vi "MegaAwesome_12_09_14b_PD(testing).vi"() -> ()   [LabVIEW 2012]
uses:
  data/MegaAwesome_States.ctl
  <vilib>/Utility/inputDevices.llb/keyboardAcquire.vi
  <vilib>/Utility/file.llb/Write To Spreadsheet File (string).vi
  <vilib>/Utility/file.llb/Read From Spreadsheet File (string).vi
panel:
  out "Vd_Sat":dbl
  in  "Vd_Sat Index":i32=2
  in  "Vd_Lin Index":i32=1
  out "Stats Label":string
  in  "Disable Flag 2":bool caption="Disable Flag"
  out "Save Next?":bool
  out "Image Center X":i32
  in  "Disable Flag":bool
  out "Index":string
  out "Opj X Axis":string
  out "X Axis Display Type":string
  in  "Index-Sat":dbl=5.0
  in  "Index-Lin":dbl=5.0
  in  "IndexLog-Lin":dbl=5.0
  in  "IndexLog-Sat":dbl=5.0 caption="Num Pts"
  out "Lin Id-Log Used":dbl[](array[numeric])
  out "Lin-Vg Array-Log Used":dbl[](array[numeric])
  out "Save Array":string[][](array[string])
  out "Folder Index":i32 caption="Length"
  out "Sat Id-Used":dbl[](array[numeric])
  out "Sat Vg Array-Used":dbl[](array[numeric])
  out "Vg Array-Log-Used":dbl[](array[numeric])
  out "Sat Id-Log-Used":dbl[](array[numeric])
  out "Lin Id-Used":dbl[](array[numeric])
  out "Lin-Vg Array-Used":dbl[](array[numeric])
  out "Lin Vd":dbl
  out "Recorded Prop":T1
  out "Current State":T2=enum."File Missing"
  in  "Main Tab Control":T3(tab)
  in  "LKG (TRF) Folder":path caption="Folder"
  out "LKG (TRF) File":path caption="File File"
  in  "Transfer File":path
  out "Transfer Folder":path
  in  "Transport\nFolder":path caption="Transport Folder"
  out "Transport\nFile":path caption="Transport File"
  in  "Image Folder":path
  out "Image File":path
  out "Fabrication Prop":T4
  out "Distances":i32[](array[numeric])
  in  "Zoom":i32(slide)=-3 scale=-5.0..5.0
  in  "Magnification":i32(ring) items=["5x", "10x", "20x", "50x", "80x"]
  in  "Undo Button":bool
  in  "Remove Button":bool
  in  "Transfer Plots":T5(tab)=enum."Saturation"
  in  "Lin-Trans Slider":dbl(slide) step=1.0 scale=0.0..61.0 scale format="%#_2p"
  out "Sqrt-Lin":cluster{dbl[], dbl[]}[](graph)
  in  "Sat-Trans Slider":dbl(slide) min=0.0 max=162.0 step=1.0 scale=0.0..61.0 scale format="%#_2p"
  out "Sqrt-Sat":cluster{dbl[], dbl[]}[](graph)
  out "Used Vg \nSqrt Sat":dbl
  out "Raw- Lin":cluster{dbl[], dbl[]}[](graph)
  out "Raw- Sat":cluster{dbl[], dbl[]}[](graph)
  in  "Log Plots":T6(tab)=enum."Saturation"
  in  "Lin-Log Slider":dbl(slide) step=1.0 scale=0.0..61.0 scale format="%#_1p"
  out "Lin-Log":cluster{dbl[], dbl[]}[](graph)
  out "Used Vg \nLog Lin":dbl
  in  "Sat-Log Slider":dbl(slide) step=1.0 scale=0.0..61.0 scale format="%#_1p"
  out "Sat-Log":cluster{dbl[], dbl[]}[](graph)
  out "Used Vg \nLog Sat":dbl
  out "Transport":cluster{ext[], ext[]}[](graph)
  out "Transport Name:":string
  out "LKG (TSF)":cluster{ext[], ext[]}[](graph)
  out "LKG (TRF) Name":string
  in  "Manual Controls":T7
  in  "File Controls":T8
  out "Date Recorded":string="Date Recorded" caption="Measured"
  out "Data Name:":string
  out "Image Name":string
  out "Date Created":string caption="Fabricated"
  in  "Comments:":string
  out "Rec: Length":dbl caption="Length"
  out "Rec: Width":dbl caption="Width"
  out "Rec: Dielectric (d)":dbl caption="Dielectric (d)" format="%#_3g"
  in  "New: Dielectric":dbl
  in  "New: Length":dbl
  in  "New: Width":dbl
  out "Rec: Temp":dbl caption="Sample Temp" format="%.1f"
  in  "New: Temp":dbl format="%.1f"
  out "Image Out":T9(plugin-control)
  in  "Num Pts":i32=5
  in  "Num Pts Log":i32=5 caption="Num Pts"
  out "Recorded Values Cluster":T10
  out "Calculated Values Cluster":T10 caption="Recorded Values Cluster"
  out "Re-Calculated Values Cluster":T10 caption="Recorded Values Cluster"
  in  "Independant Variable:":string(combo)="Length (um):"
  out "Image Preview":T9(plugin-control)
  out "Total Width":i32
  in  "Index Array":i32(ring) caption="Index" items=["2M", "2N", "2O", "2P", "3M", "3N", "3O", "3P"]
  in  "Hysteresis Analysis":enum32{"1st Sweep", "2nd Sweep", "Both"}(radio)
  in  "Dielectric Constant":dbl=3.9
  in  "Scale Factors":T11={"5x"=0.5495, "10x"=0.2755, "20x"=0.1389, "50x"=0.0546, "80x"=0.0337}
  in  "Room Temp":dbl=294.0 caption="Room Temp (K)"
  out "No Image\n File":path=path "\\\\acad1\\physics/Jurchescu-group/JW-PD/Mega Awesome/data/Image Not Found.png" caption="No Image File"
  out "Origin Project File":path=path "\\\\acad1\\physics/Jurchescu-group/JW-PD/Mega Awesome/data/Origin Template.opj"
  out "No Transport\n File":path=path "\\\\acad1\\physics/Jurchescu-group/JW-PD/Mega Awesome/data/No Transport File.txt" caption="No Transport File"
  in  "Transport Style Controls":T12={"Transport Line Size"=1, "Transport Line Color"=16772608} {"Transport Line Size" items=["Extra Small", "Small", "Medium", "Large", "Extra Large"]}
  out "Application Directory":path=path "\\\\acad1\\physics/Jurchescu-group/JW-PD/Mega Awesome"
  in  "LKG Style Controls":T13={"Transport Line Size"=1, "LKG (TRF) Line Color"=16772608} {"Transport Line Size" items=["Extra Small", "Small", "Medium", "Large", "Extra Large"]}
  out "Progress":i32(slide) max=46 step=1 scale=0.0..100.0
  # "1)  Select the Transfer File that you would like to analyze:"
  # "Transfer Location"
  # "2) What else would you like to view during your analysis?"
  # "Transport Location"
  # "Image Location"
  # "Gate Leakge (TRF) Location"
  # "Recorded"
  # "Calculated"
  # "Re-Calculated"
  # "Manual"
  # "um"
  # "V"
  # "V"
  # "V"
  # "Default File Choices"
  # "Scale Factors"
  # "Default Analysis Values"
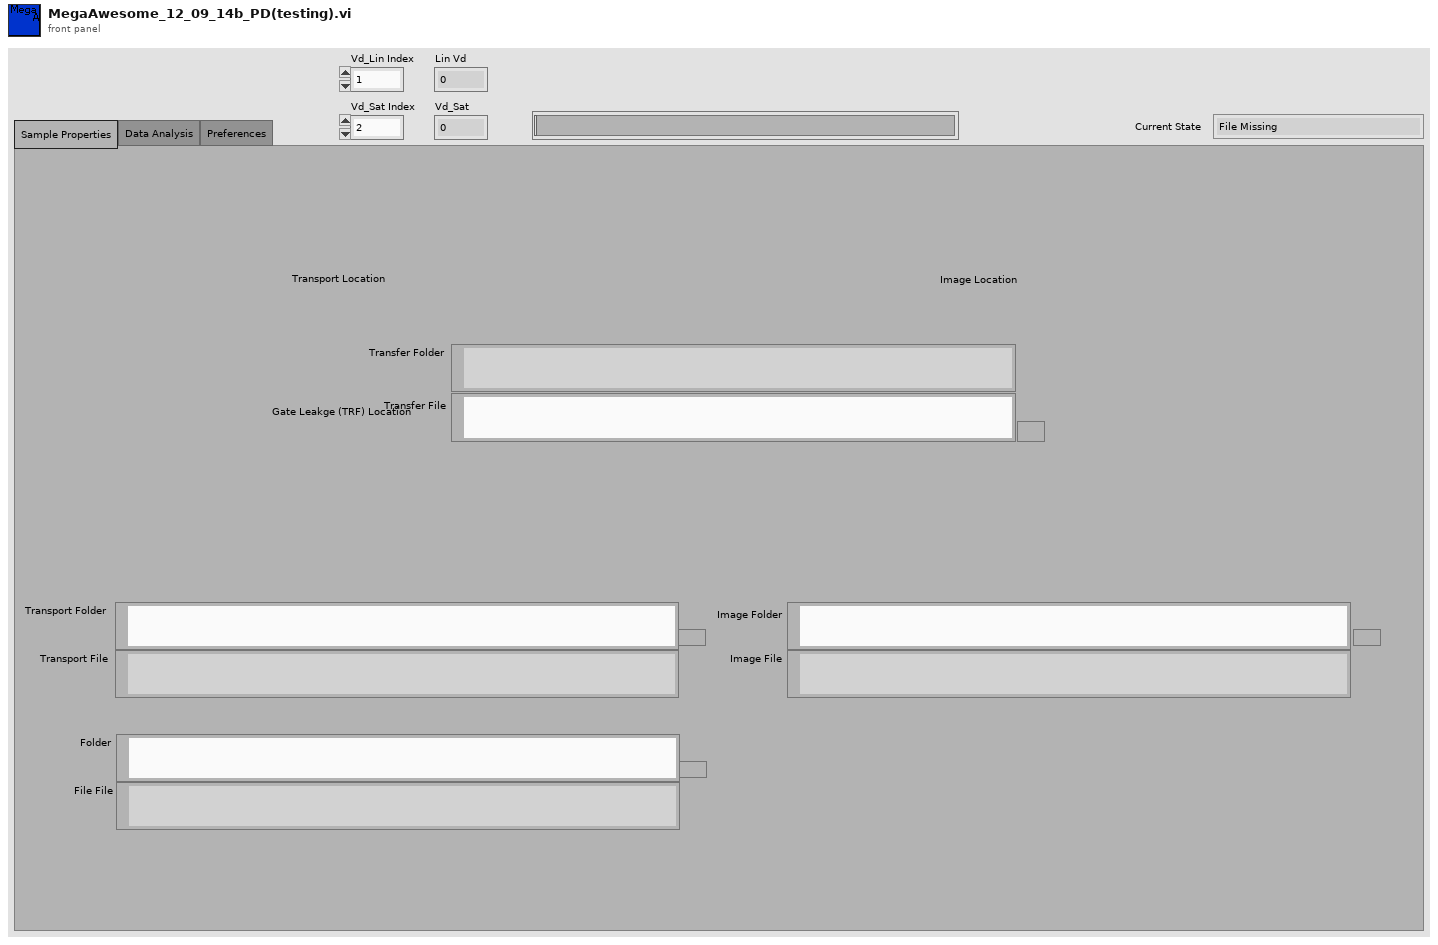
[diagram p1: front panel]
types:
  T1 = cluster{"Date Recorded":string, "Index":string, "Length":dbl, "Width":dbl, "Sample Temp":dbl}
  T2 = typedef "MegaAwesome_States.ctl" = enum16{"Init", "File Missing", "No Event", "Read Data", "Calculated Values", "Re-Calculated Values", "Next File", "Previous File", "Discard File", "Save", "Save Lines", "Export", "Exit"}
  T3 = enum32{"Sample Properties", "Data Analysis", "Preferences"}
  T4 = cluster{"Date Created":string, "Material":string, "Solvent":string, "Concentration":dbl, "Method":string, "Dielectric (nm)":dbl, "Treatment":string, "Comments":string}
  T5 = enum32{"Linear", "Saturation", "Raw-Linear", "Raw-Saturation"}
  T6 = enum32{"Linear", "Saturation", "Transport", "Gate Current (TSF)"}
  T7 = cluster{"Manual-Temp":bool, "Manual-Width":bool, "Manuel-Length":bool, "Manuel-Dielectric":bool, "Manual Comments":bool}
  T8 = cluster{"Previous File":bool, "Discard ":bool, "Save Lines":bool, "Close":bool, "Next File ":bool, "Save":bool, "Save Next":bool, "Export":bool}
  T9 = typedef "IMAQ Image.ctl" = refnum<image>
  T10 = cluster{"Mobility-Sat":dbl, "Moblitity-Lin":dbl, "On/Off":dbl, "Off Current":dbl, "Vt-Sat":dbl, "STS":dbl, "Trap Density-VT":dbl, "Trap Density-STS":dbl}
  T11 = cluster{"5x":dbl, "10x":dbl, "20x":dbl, "50x":dbl, "80x":dbl}
  T12 = cluster{"Transport Line Size":u16, "Transport Line Color":u32}
  T13 = cluster{"Transport Line Size":u16, "LKG (TRF) Line Color":u32}
  T14 = enum8{"Enabled", "Disabled", "Disabled and Grayed Out"}
  T15 = typedef "LVBoundsTypeDef.ctl" = cluster{"Width":u32, "Height":u32}
  T16 = enum16{"0", "1", "2", "3", "4", "5", "6", "7", "8", "9", "A", "B", "C", "D", "E", "F", "G", "H", "I", "J", "K", "L", "M", "N", "O", "P", "Q", "R", "S", "T", "U", "V", "W", "X", "Y", "Z", "F1", "F2", "F3", "F4", "F5", "F6", "F7", "F8", "F9", "F10", "F11", "F12", "F13", "F14", "F15", "ADD", "BACK", "BACKSLASH", "CAPITAL", "COMMA", "DECIMAL", "DELETE", "DIVIDE", "DOWN", "END", "EQUALS", "ESCAPE", "GRAVE (`)", "HOME", "INSERT", "LBRACKET", "LCONTROL", "LEFT", "L ALT", "LSHIFT", "LWIN", "MINUS", "MULTIPLY", "NEXT", "NUMLOCK", "NUMPAD_0", "NUMPAD_1", "NUMPAD_2", "NUMPAD_3", "NUMPAD_4", "NUMPAD_5", "NUMPAD_6", "NUMPAD_7", "NUMPAD_8", "NUMPAD_9", "PAUSE", "PERIOD", "PRIOR (PG UP)", "RBRACKET", "RCONTROL", "RETURN", "RIGHT", "R ALT", "RSHIFT", "RWIN", "SCROLL", "SEMICOLON", "SLASH", "SPACE", "SUBTRACT", "TAB", "UP", "ENTER (num pad)", "' (quote)"}[]
  T17 = enum16{"0", "1", "2", "3", "4", "5", "6", "7", "8", "9", "A", "B", "C", "D", "E", "F", "G", "H", "I", "J", "K", "L", "M", "N", "O", "P", "Q", "R", "S", "T", "U", "V", "W", "X", "Y", "Z", "F1", "F2", "F3", "F4", "F5", "F6", "F7", "F8", "F9", "F10", "F11", "F12", "F13", "F14", "F15", "ADD", "BACK", "BACKSLASH", "CAPITAL", "COMMA", "DECIMAL", "DELETE", "DIVIDE", "DOWN", "END", "EQUALS", "ESCAPE", "GRAVE (`)", "HOME", "INSERT", "LBRACKET", "LCONTROL", "LEFT", "L ALT", "LSHIFT", "LWIN", "MINUS", "MULTIPLY", "NEXT", "NUMLOCK", "NUMPAD_0", "NUMPAD_1", "NUMPAD_2", "NUMPAD_3", "NUMPAD_4", "NUMPAD_5", "NUMPAD_6", "NUMPAD_7", "NUMPAD_8", "NUMPAD_9", "PAUSE", "PERIOD", "PRIOR (PG UP)", "RBRACKET", "RCONTROL", "RETURN", "RIGHT", "R ALT", "RSHIFT", "RWIN", "SCROLL", "SEMICOLON", "SLASH", "SPACE", "SUBTRACT", "TAB", "UP", "ENTER (num pad)", "' (quote)"}
  T18 = typedef "ROI Descriptor" = cluster{"Global Rectangle":i32[], "Contours":cluster{"ID":enum32{"External", "Internal"}, "Type":u32, "Coordinates":i32[]}[]}
  T19 = cluster{string, sgl, bool, bool, bool, bool, bool, bool, i32}
  T20 = cluster{i32, cluster{string, sgl, bool, bool, bool, bool, bool, bool, i32}, i32, i32}
  T21 = cluster{"Global Rectangle":i32[], "Contours":cluster{"Contour Type":u32, "ROI Type":u32, "Points":i32[]}[]}
  T22 = cluster{"Contour Type":u32, "ROI Type":u32, "Points":i32[]}[]
  T23 = cluster{"[0]":cluster{dbl[], dbl[]}, "[1]":cluster{dbl[], dbl[]}, "[2]":cluster{dbl[], dbl[]}, "[3]":cluster{dbl[], dbl[]}, "[4]":cluster{dbl[], dbl[]}, "[5]":cluster{dbl[], dbl[]}, "[6]":cluster{dbl[], dbl[]}, "[7]":cluster{dbl[], dbl[]}, "[8]":cluster{dbl[], dbl[]}}
  T24 = cluster{i32[], cluster{"Contour Type":u32, "ROI Type":u32, "Points":i32[]}[]}
  T25 = cluster{"Contour Type":u32, "ROI Type":u32, "Points":i32[]}
  T26 = cluster{"Points[0]":i32, "Points[1]":i32, "Points[2]":i32, "Points[3]":i32, "Points[4]":i32, "Points[5]":i32, "Points[6]":i32, "Points[7]":i32, "Points[8]":i32}
  T27 = cluster{"Sat Vg Used":dbl[], "Sat Sqrt(Id) Used ":dbl[], "Lin Vg Used":dbl[], "Lin Sqrt(Id) Used":dbl[], "Index-Lin":dbl, "Index-Sat":dbl}
  T28 = cluster{"Raw Sat":cluster{dbl[], dbl[]}[], "Sqrt Sat":cluster{dbl[], dbl[]}[], "Log Sat":cluster{dbl[], dbl[]}[], "Raw Lin":cluster{dbl[], dbl[]}[], "Sqrt Lin":cluster{dbl[], dbl[]}[], "Log Lin":cluster{dbl[], dbl[]}[]}
  T29 = cluster{"Mobility-Sat":dbl, "Vt-Sat":dbl, "Mobility-Lin":dbl, "Vt-Lin":dbl, "Off I-Sat":dbl, "On/Off I-Sat":dbl}
  T30 = cluster{"Sat Vg Used":dbl[], "Sat Log(Id) Used":dbl[], "Lin Vg Used":dbl[], "Lin Log(Id) Used":dbl[], "STS Index-Sat":dbl, "STS Index-Lin":dbl}
  T31 = cluster{"Independant  Variable Indicator":string, "Parameter String Indicator":string}
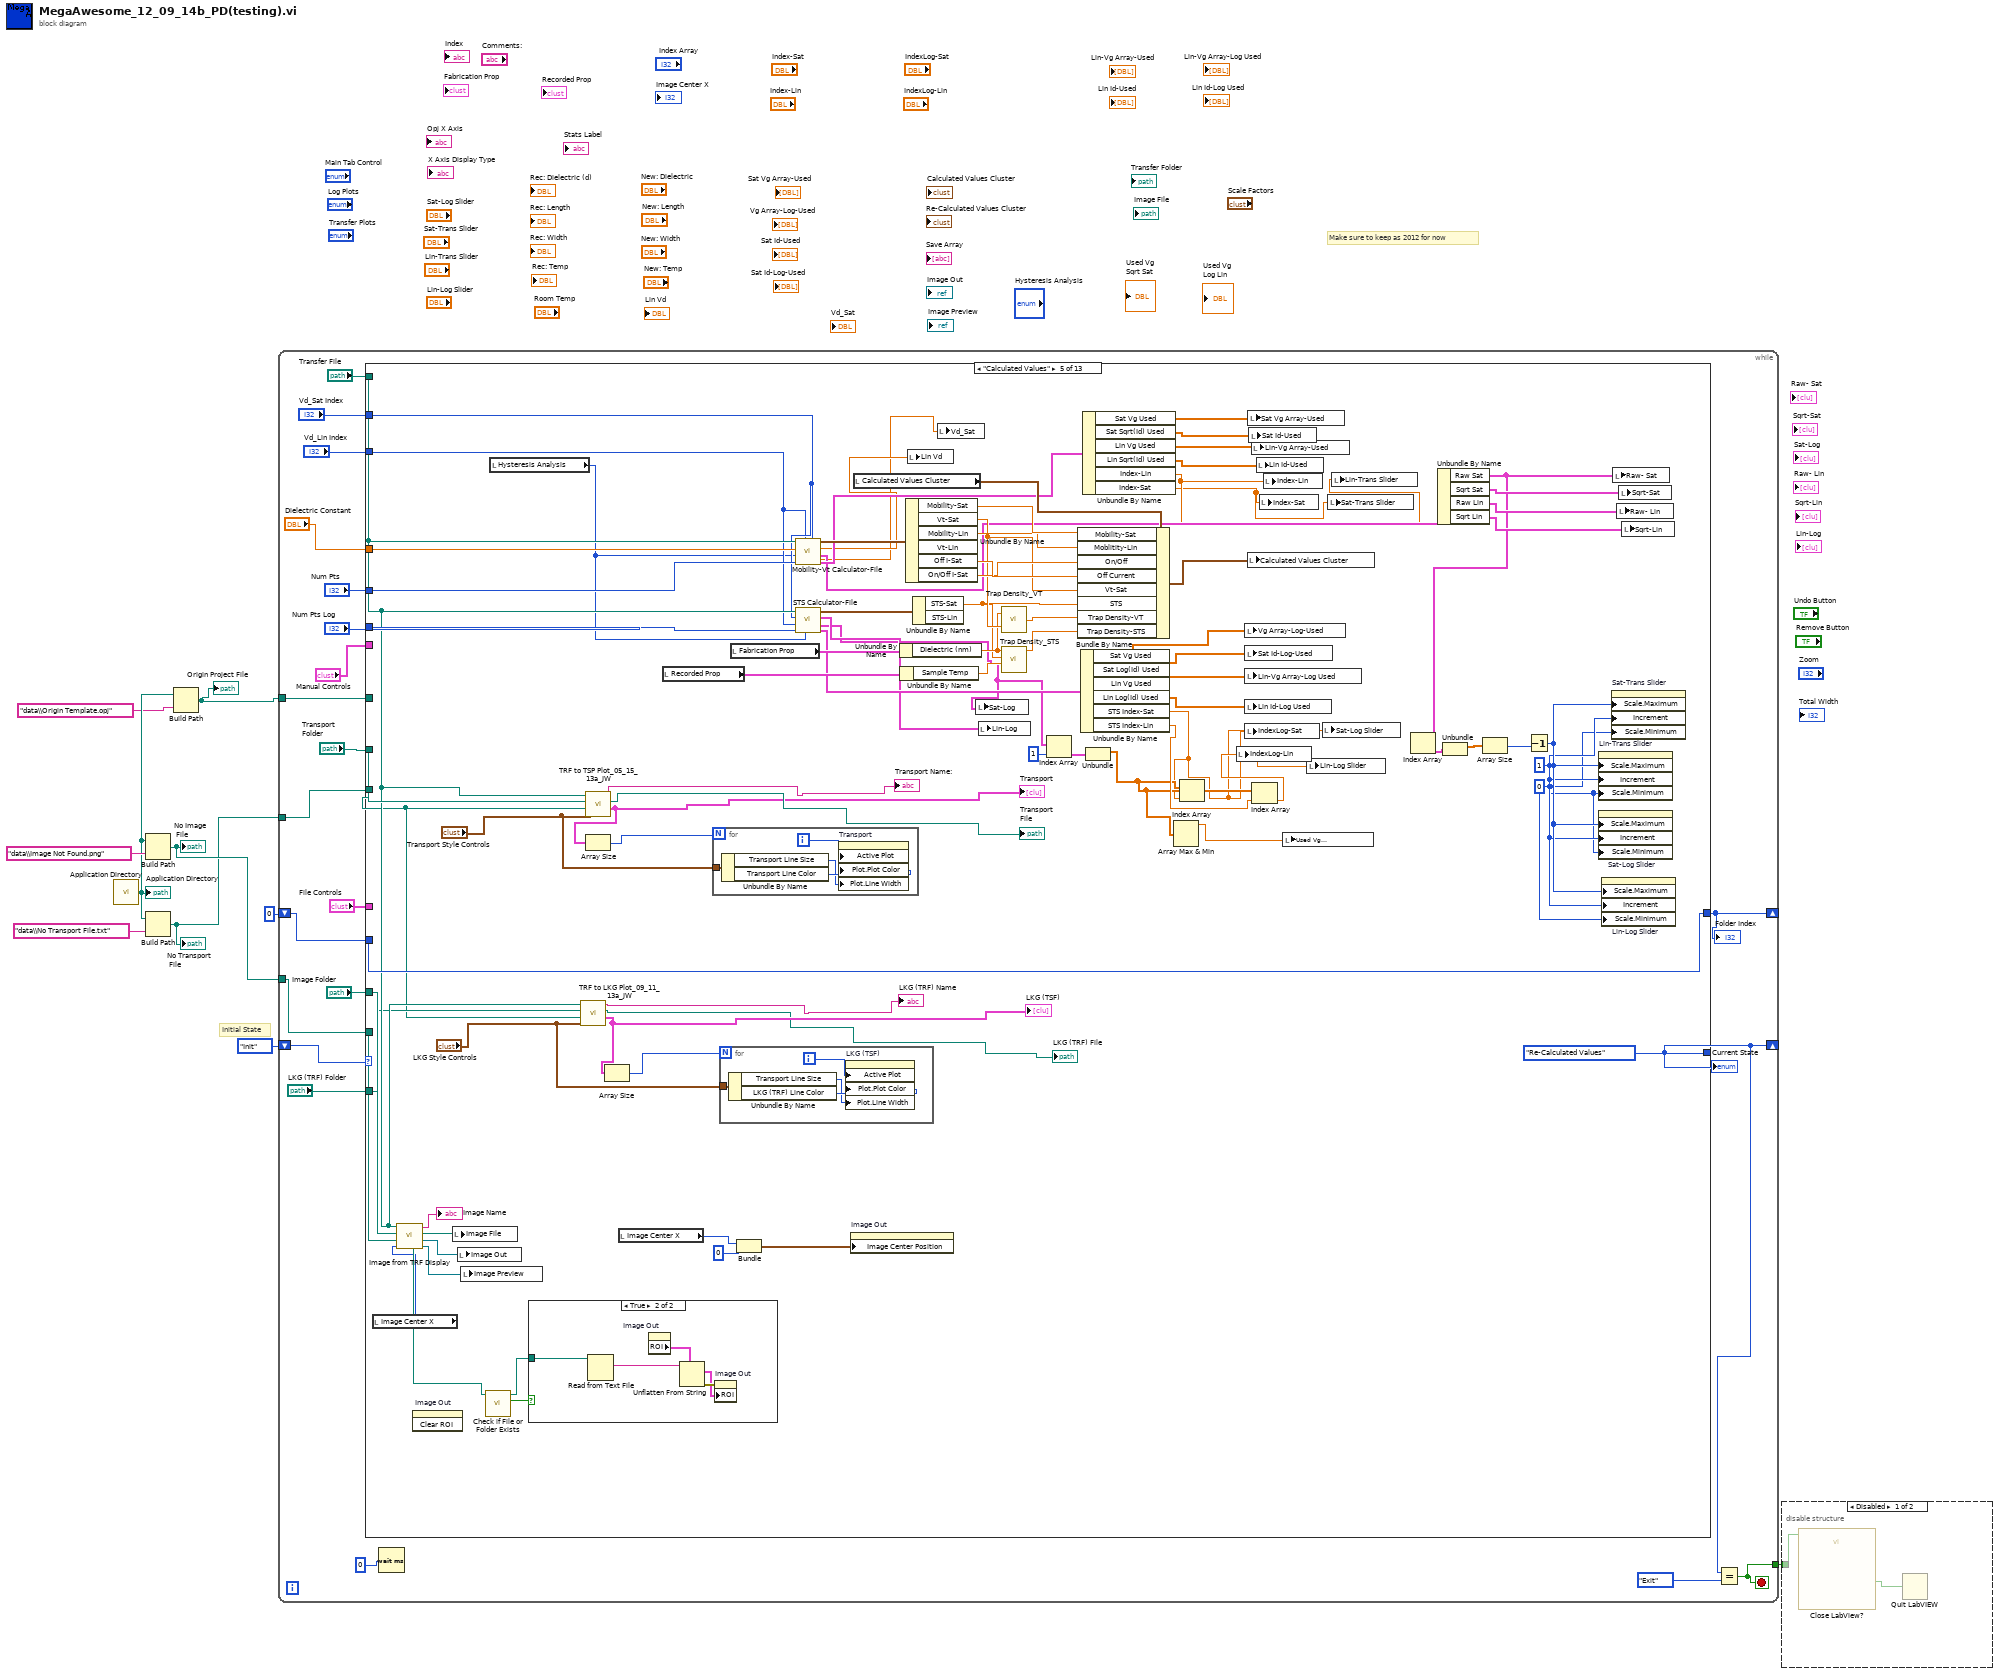
[diagram p0: block diagram]
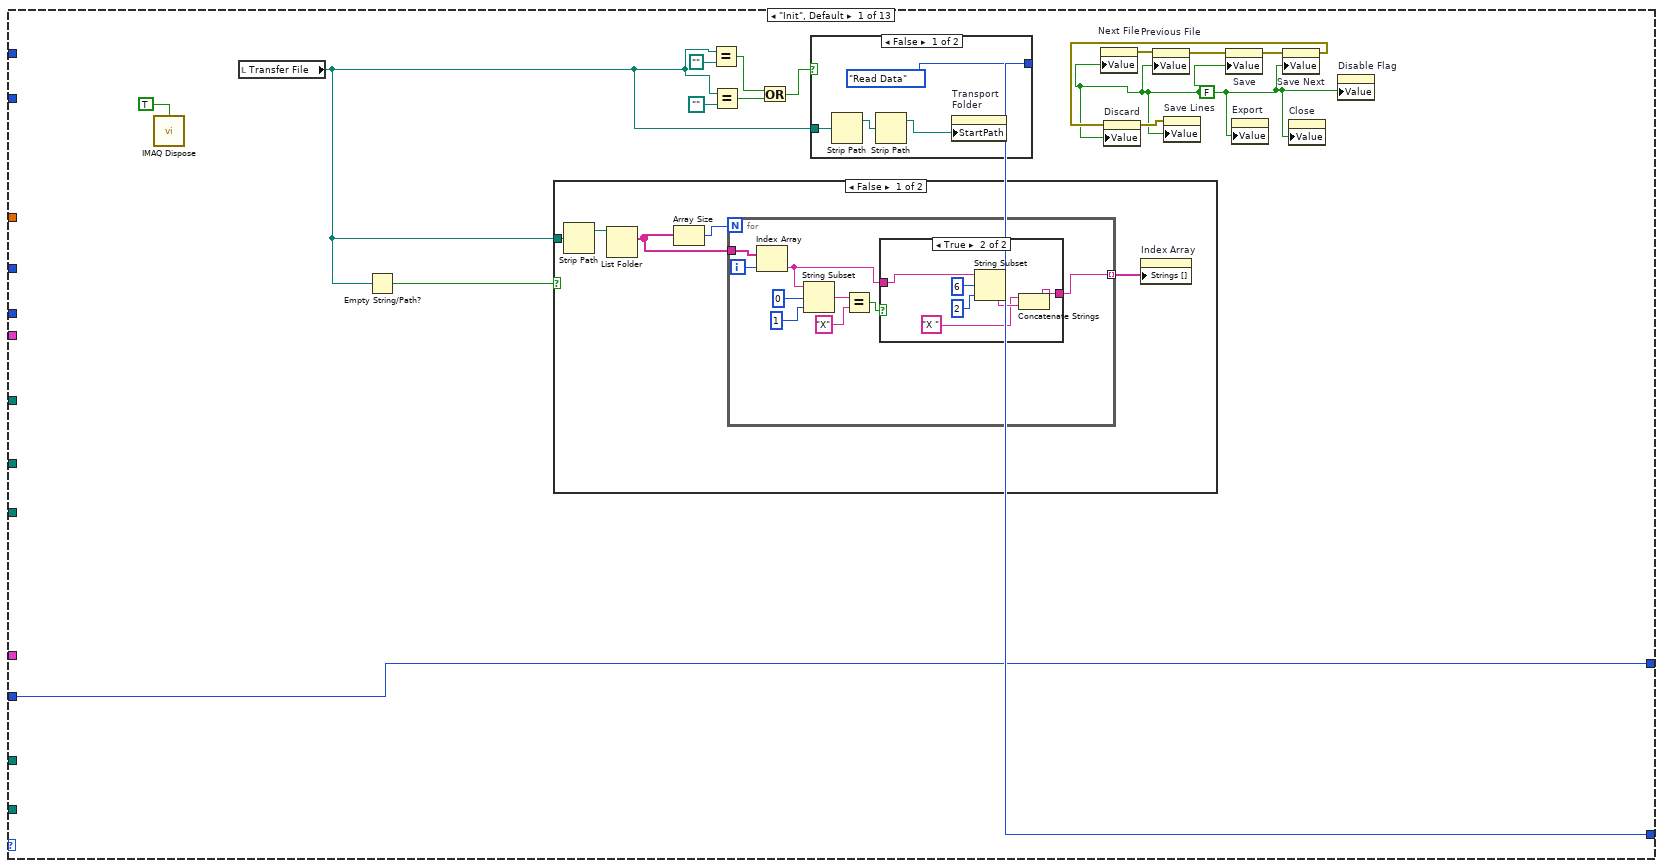
[diagram p3: hidden frame]
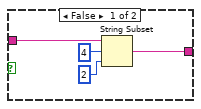
[diagram p4: hidden frame]
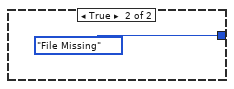
[diagram p6: hidden frame]
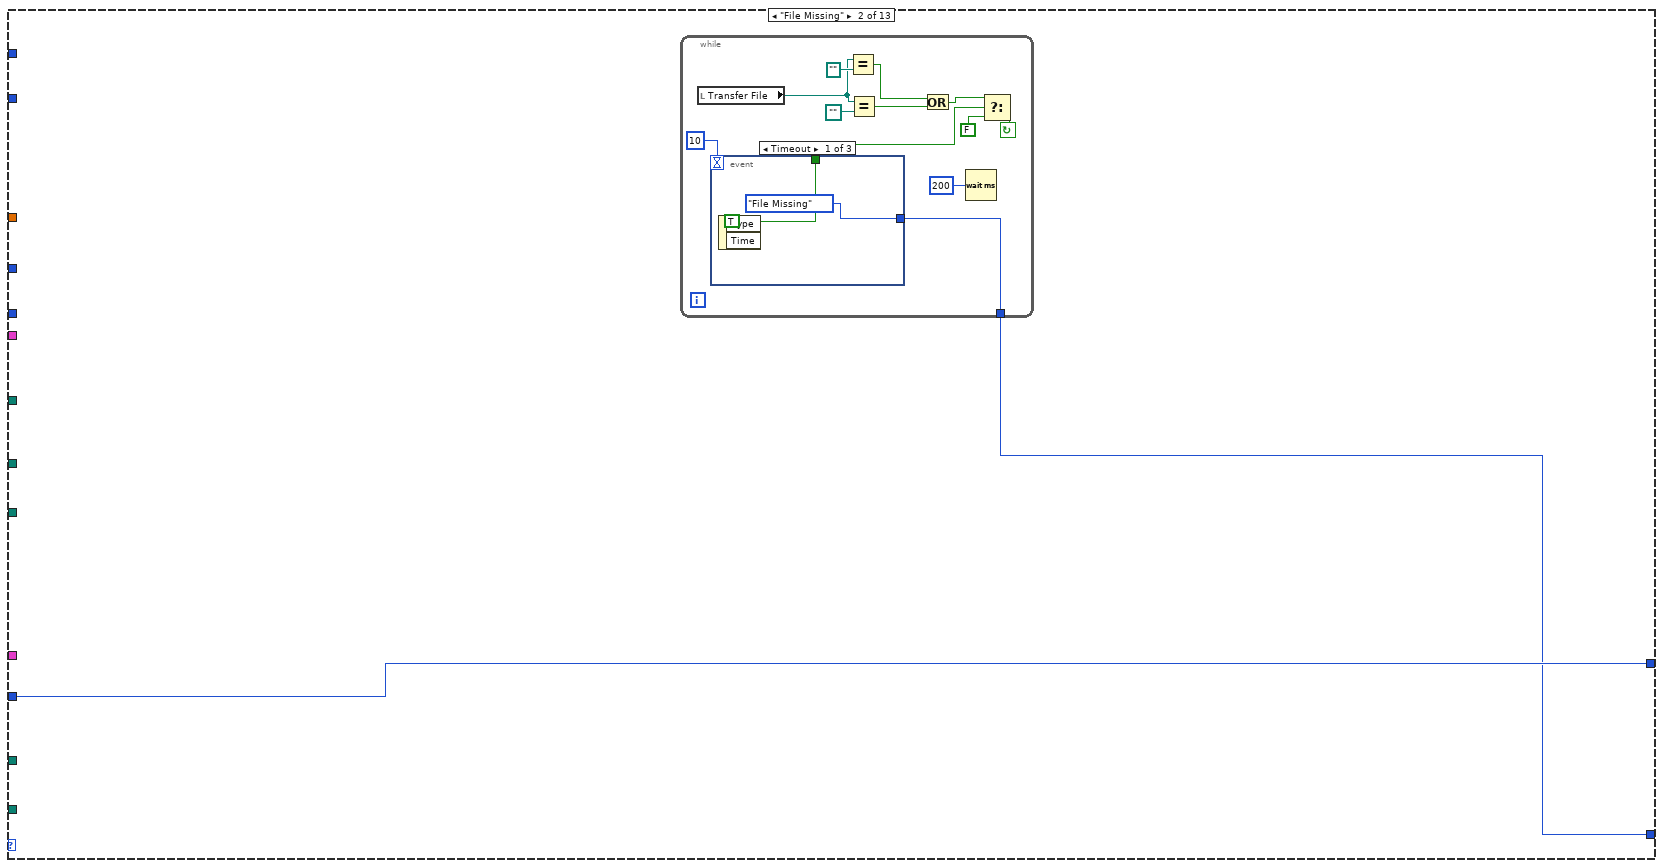
[diagram p7: hidden frame]
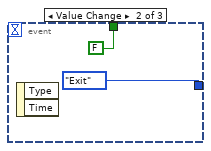
[diagram p8: hidden frame]
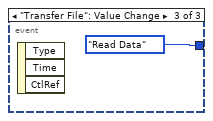
[diagram p9: hidden frame]
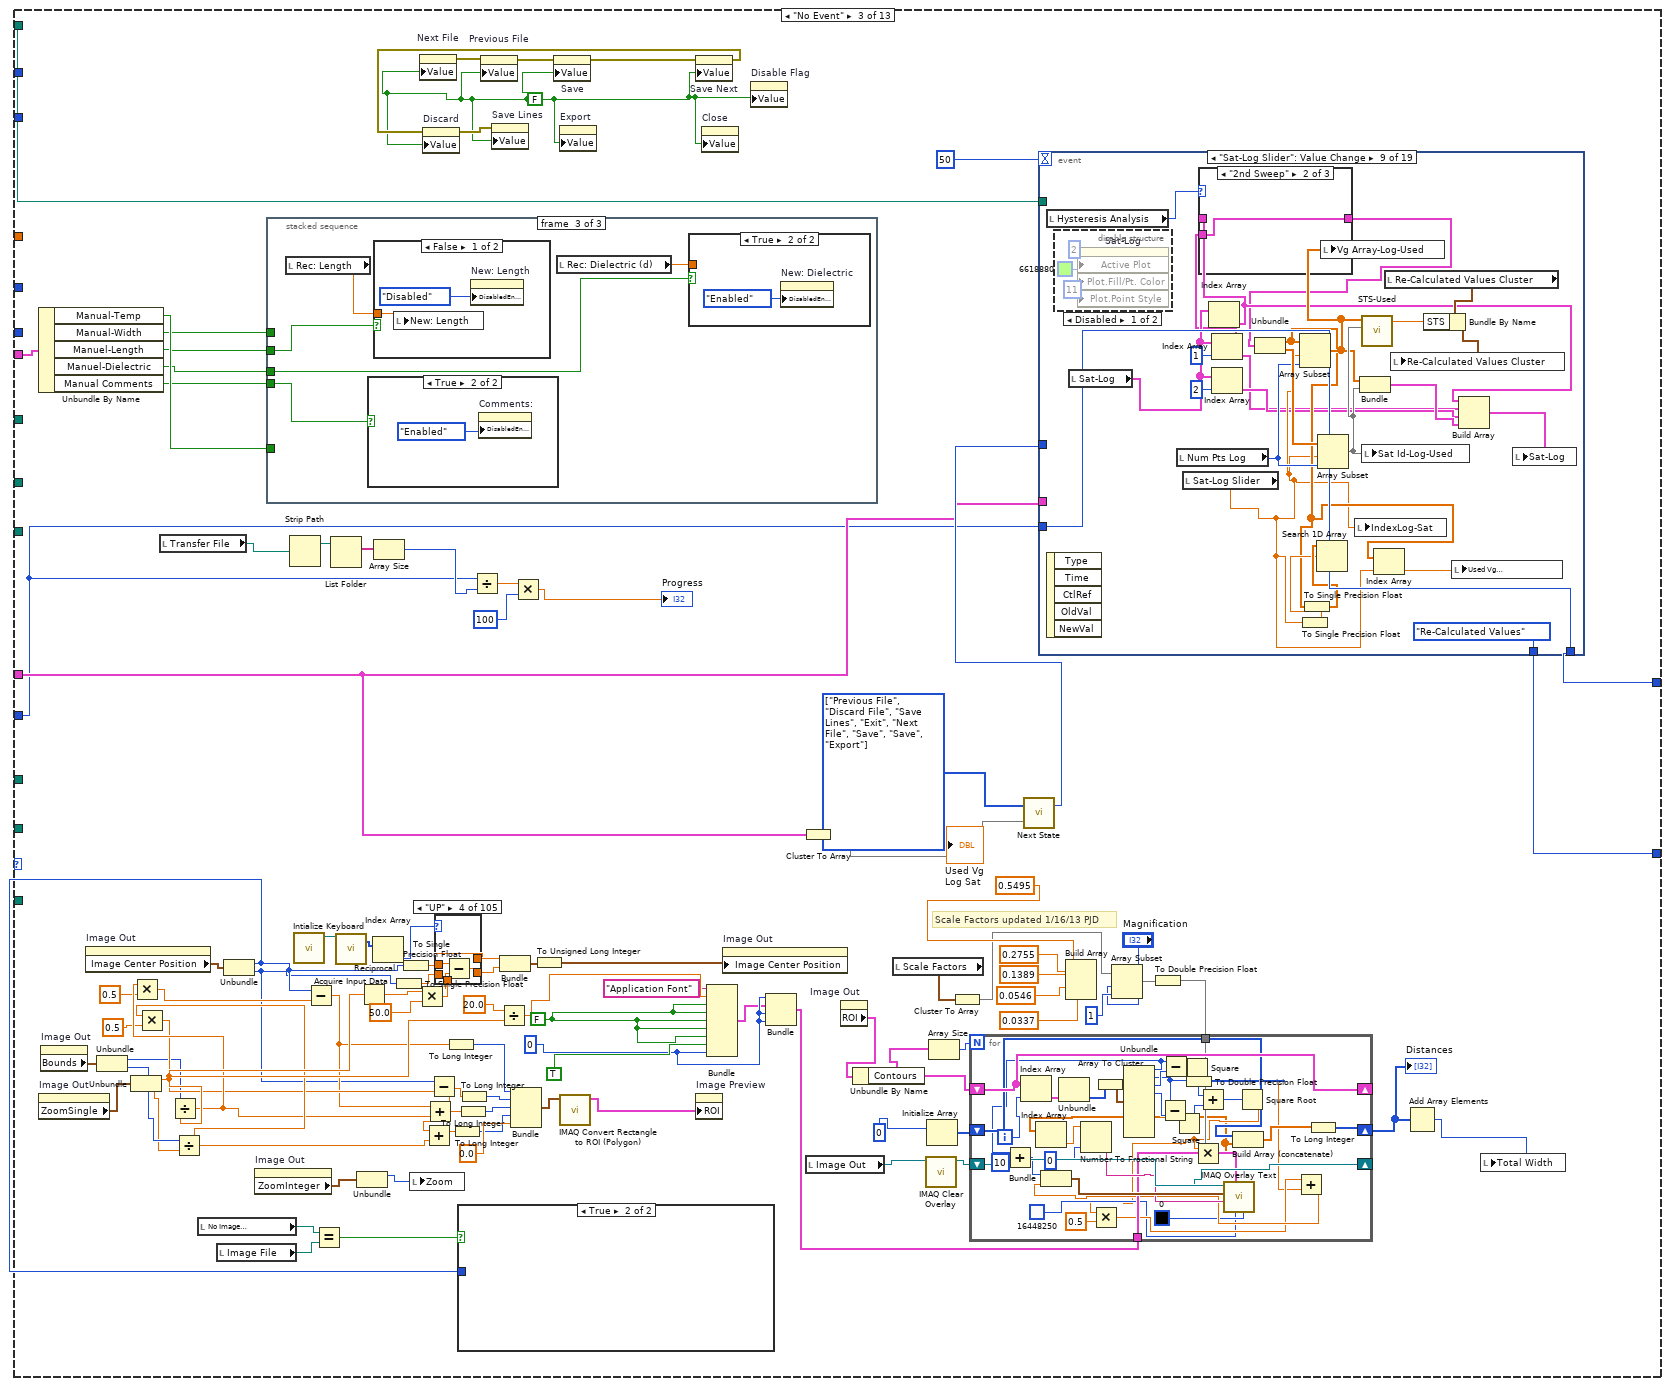
[diagram p10: hidden frame]
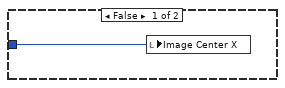
[diagram p11: hidden frame]
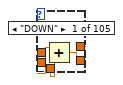
[diagram p12: hidden frame]
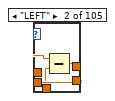
[diagram p13: hidden frame]
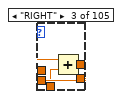
[diagram p14: hidden frame]
diagram:
  # "Make sure to keep as 2012 for now"
  # "Initial State"
  n1 = call <vilib>:"Application Directory.vi"() -> ("Application Directory"=w4:path)
  "Application Directory" <- w4
  n2 = Build Path(base path=w4, name or relative path="data\\Image Not Found.png") -> (appended path=w6:path)
  "No Image\n File" <- w6
  n3 = Build Path(base path=w4, name or relative path="data\\No Transport File.txt") -> (appended path=w5:path)
  "No Transport\n File" <- w5
  n4 = Build Path(base path=w4, name or relative path="data\\Origin Template.opj") -> (appended path=w1:path)
  "Origin Project File" <- w1
  n5 = while {
    shift-right: [w17] -> _
    shift-left: MegaAwesome_States."Init" -> [w19]
    shift-right: [w16] -> _
    shift-left: 0 -> [w26]
    tunnel: w6 -> [w23]
    tunnel: w5 -> [w21]
    tunnel: [w20] -> w2
    tunnel: w1 -> [w13]
    stop <- w20 stop-if-true
    n6 = case shown="\"Calculated Values\"" w19 {
      tunnel: [w34 w77 w185 MegaAwesome_States."Calculated Values" MegaAwesome_States."Re-Calculated Values" MegaAwesome_States."No Event" MegaAwesome_States."Read Data" MegaAwesome_States."Read Data" MegaAwesome_States."Init" w919 MegaAwesome_States."Exit" MegaAwesome_States."No Event" MegaAwesome_States."No Event"] -> w17
      tunnel: "Transfer File" -> [_ _ w96 w683 w746 _ w858 w869 w896 w913 _ _ _]
      tunnel: "Num Pts" -> [_ _ _ _ w787 _ _ _ _ _ _ _ _]
      tunnel: "Num Pts Log" -> [_ _ _ _ w786 _ _ _ _ _ _ _ _]
      tunnel: "Image Folder" -> [_ _ _ _ w783 _ _ _ _ _ _ w1430 _]
      tunnel: w23 -> [_ _ _ _ w782 _ _ _ _ _ _ _ _]
      tunnel: [w32 w78 w178 w687 w781 w818 w844 w867 w885 w920 w1416 w1440 w1446] -> w16
      tunnel: w26 -> [w32 w78 w99 w676 w781 w818 w845 w868 _ w920 w1416 w1440 w1446]
      tunnel: "Manual Controls" -> [_ _ w187 w674 _ _ _ _ _ _ _ _ _]
      tunnel: "File Controls" -> [_ _ w176 _ _ _ _ _ _ _ _ _ _]
      tunnel: "Transport\nFolder" -> [_ _ _ _ w758 _ _ _ _ _ _ _ _]
      tunnel: w21 -> [_ _ _ _ w744 _ _ _ _ _ _ _ _]
      tunnel: "LKG (TRF) Folder" -> [_ _ _ w675 w745 _ _ _ _ _ _ _ _]
      tunnel: "Dielectric Constant" -> [_ _ _ _ w738 w816 _ _ _ _ _ _ _]
      tunnel: w13 -> [_ _ _ _ _ _ _ _ _ _ _ _ w1444]
      tunnel: "Vd_Lin Index" -> [_ _ _ _ w735 _ _ _ _ _ _ _ _]
      tunnel: "Vd_Sat Index" -> [_ _ _ _ w736 _ _ _ _ _ _ _ _]
      frame "Init", Default {
        w35 = FALSE
        n7 = call "IMAQ Dispose"("All Images? (No)"=TRUE) -> ()  [unwired: 5 in, 1 out]
        n8 = local read "Transfer File"() -> (w33:path)
        n9 = Empty String/Path?(string/path=w33) -> (empty?=w42:bool)
        n10 = case shown="False" w42 {
          tunnel: w33 -> [w49 _]
          frame False {
            n11 = Strip Path(path=w49) -> (stripped path=w51:path)  [unwired: 1 out]
            n12 = List Folder(path=w51) -> (filenames=w50:string[])  [unwired: 3 in, 3 out]
            n13 = Array Size(array=w50) -> (size(s)=w52:i32)
            n14 = for {
              N: w52 -> [_]
              tunnel: w50 -> [w61]
              tunnel: [w59] -> w48 mode=indexing
              i -> [w60]
              n15 = Index Array(array=w61, index=w60) -> (element=w58:string)
              n16 = String Subset(string=w58, offset (0)=0, length (rest)=1) -> (substring=w55:string)
              n17 = Equal?(x=w55, y="X") -> (x = y?=w54:bool)
              n18 = case shown="True" w54 {
                tunnel: w58 -> [w65 w69]
                tunnel: [w62 w68] -> w59
                frame False {
                  n19 = String Subset(string=w65, offset (0)=4, length (rest)=2) -> (substring=w62:string)
                }
                frame True {
                  n20 = String Subset(string=w69, offset (0)=6, length (rest)=2) -> (substring=w67:string)
                  n21 = Concatenate Strings("X ", w67) -> (w68:string)
                }
              }
            }
            n22 = property on="Index Array" class="Ring (strict)"("Strings []"=w48) -> ()  [unwired: 2 in, 2 out]
          }
          frame True {
          }
        }
        n23 = Equal?(x=w33, y=path "") -> (x = y?=w45:bool)
        n24 = Equal?(x=w33, y=path "") -> (x = y?=w44:bool)
        n25 = Or(x=w45, y=w44) -> (x .or. y?=w47:bool)
        n26 = case shown="False" w47 {
          tunnel: [MegaAwesome_States."Read Data" MegaAwesome_States."File Missing"] -> w34
          tunnel: w33 -> [w74 _]
          frame False {
            n27 = Strip Path(path=w74) -> (stripped path=w73:path)  [unwired: 1 out]
            n28 = Strip Path(path=w73) -> (stripped path=w72:path)  [unwired: 1 out]
            n29 = property on="Transport\nFolder" class="Path"("StartPath"=w72) -> ()  [unwired: 2 in, 2 out]
          }
          frame True {
          }
        }
        n30 = property on="Next File" class="Bool (strict)"("Value"=w35) -> (error out=w40:errorcluster)  [unwired: 2 in, 1 out]
        n31 = property on="Previous File" class="Bool (strict)"(error in=w40, "Value"=w35) -> (error out=w39:errorcluster)  [unwired: 1 in, 1 out]
        n32 = property on="Save" class="Bool (strict)"(error in=w39, "Value"=w35) -> (error out=w38:errorcluster)  [unwired: 1 in, 1 out]
        n33 = property on="Export" class="Bool (strict)"("Value"=w35) -> ()  [unwired: 2 in, 2 out]
        n34 = property on="Save Next" class="Bool (strict)"(error in=w38, "Value"=w35) -> (error out=w37:errorcluster)  [unwired: 1 in, 1 out]
        n35 = property on="Discard" class="Bool (strict)"(error in=w37, "Value"=w35) -> (error out=w36:errorcluster)  [unwired: 1 in, 1 out]
        n36 = property on="Save Lines" class="Bool (strict)"(error in=w36, "Value"=w35) -> ()  [unwired: 1 in, 2 out]
        n37 = property on="Close" class="Bool (strict)"("Value"=w35) -> ()  [unwired: 2 in, 2 out]
        n38 = property on="Disable Flag" class="Bool (strict)"("Value"=w35) -> ()  [unwired: 2 in, 2 out]
      }
      frame "File Missing" {
        n39 = while {
          tunnel: [w85] -> w77
          stop <- w81 continue-if-true
          n40 = local read "Transfer File"() -> (w86:path)
          n41 = event shown="[0] Timeout" {
            selector: _ -> [_ _ _]
            dyn-events: _ -> [_ _ _]
            timeout: 10 -> [_ _ _]
            tunnel: [MegaAwesome_States."File Missing" MegaAwesome_States."Exit" MegaAwesome_States."Read Data"] -> w85
            tunnel: [TRUE FALSE _] -> w84
            event Timeout {
              n42 = event-data() -> ()  [unwired: 1 in, 2 out]
            }
            event "File Controls.Close": Value Change {
              n43 = event-data() -> ()  [unwired: 1 in, 2 out]
            }
            event "Transfer File": Value Change {
              n44 = event-data() -> ()  [unwired: 1 in, 3 out]
            }
          }
          n45 = Equal?(x=w86, y=path "") -> (x = y?=w88:bool)
          n46 = Equal?(x=w86, y=path "") -> (x = y?=w89:bool)
          n47 = Or(x=w88, y=w89) -> (x .or. y?=w83:bool)
          n48 = Wait (ms)(milliseconds to wait=u32 200) -> ()  [unwired: 1 out]
          n49 = Select(t=w83, s=w84, f=FALSE) -> (s? t:f=w81:bool)
        }
      }
      frame "No Event" {
        w167 = FALSE
        w169 = 0
        w177 = FALSE
        w194 = T2[] [enum."Previous File", enum."Discard File", enum."Save Lines", enum."Exit", enum."Next File", enum."Save", enum."Save", enum."Export"] items=["Init", "File Missing", "No Event", "Read Data", "Calculated Values", "Re-Calculated Values", "Next File", "Previous File", "Discard File", "Save", "Save Lines", "Export", "Exit"]
        # "Scale Factors updated 1/16/13 PJD"
        n50 = Unbundle By Name(w187) -> ("Manual-Temp"=w192:bool, "Manual-Width"=w191:bool, "Manuel-Length"=w190:bool, "Manuel-Dielectric"=w189:bool, "Manual Comments"=w188:bool)
        n51 = property on="Image Out" class="ImageControl"() -> ("ZoomSingle"=w156:cluster{"X":sgl, "Y":sgl})  [unwired: 2 in, 2 out]
        n52 = property on="Image Out" class="ImageControl"() -> ("Bounds"=w155:T15)  [unwired: 2 in, 2 out]
        n53 = property on="Image Out" class="ImageControl"() -> ("Image Center Position"=w152:cluster{"X":u32, "Y":u32})  [unwired: 2 in, 2 out]
        n54 = Unbundle(w155) -> ("Width"=w158:u32, "Height"=w159:u32)
        n55 = Unbundle(w156) -> ("X"=w173:sgl, "Y"=w157:sgl)
        n56 = local read "Transfer File"() -> (w102:path)
        n57 = Divide(x=w158, y=w173) -> (x/y=w164:sgl)
        n58 = Multiply(x=w164, y=sgl 0.5) -> (x*y=w162:sgl)
        n59 = Divide(x=w159, y=w157) -> (x/y=w165:sgl)
        n60 = Multiply(x=w165, y=sgl 0.5) -> (x*y=w163:sgl)
        n61 = local read "No Image\n File"() -> (w127:path)
        n62 = local read "Image File"() -> (w126:path)
        n63 = Unbundle(w152) -> ("X"=w109:u32, "Y"=w107:u32)
        n64 = property on="Image Out" class="ImageControl"() -> ("ZoomInteger"=w130:cluster{"X":i32, "Y":i32})  [unwired: 2 in, 2 out]
        n65 = stacked-sequence {
          tunnel: w192 -> [w627 _ _]
          tunnel: w191 -> [_ w641 _]
          tunnel: w190 -> [_ _ w654]
          tunnel: w189 -> [_ _ w652]
          tunnel: w188 -> [_ _ w651]
          frame #0 {
            n66 = local read "Rec: Temp"() -> (w626:dbl)
            n67 = case shown="True" w627 {
              tunnel: w626 -> [w632 _]
              frame False {
                n68 = local read "Rec: Temp"() -> (w630:dbl)
                n69 = property on="New: Temp" class="DigNum (strict)"("DisabledEnum"=T14."Disabled" ("Disabled")) -> ()  [unwired: 2 in, 2 out]
                n70 = Equal To 0?(x=w630) -> (x = 0?=w631:bool)
                n71 = local write "New: Temp"(w632) -> ()
                n72 = case shown="True" w631 {
                  tunnel: [w633 w634] -> w628
                  tunnel: w630 -> [w633 _]
                  frame False {
                  }
                  frame True {
                    n73 = local read "Room Temp"() -> (w634:dbl)
                  }
                }
                n74 = local write "Rec: Temp"(w628) -> ()
                n75 = local write "New: Temp"(w628) -> ()
              }
              frame True {
                n76 = property on="New: Temp" class="DigNum (strict)"("DisabledEnum"=T14."Enabled" ("Disabled")) -> ()  [unwired: 2 in, 2 out]
              }
            }
          }
          frame #1 {
            n77 = local read "New: Width"() -> (w642:dbl)
            n78 = local read "Total Width"() -> (w638:i32)
            n79 = case shown="True" w641 {
              frame False {
                n80 = property on="New: Width" class="DigNum (strict)"("DisabledEnum"=T14."Disabled" ("Disabled")) -> ()  [unwired: 2 in, 2 out]
              }
              frame True {
                n81 = property on="New: Width" class="DigNum (strict)"("DisabledEnum"=T14."Enabled" ("Disabled")) -> ()  [unwired: 2 in, 2 out]
              }
            }
            n82 = Not(x=w641) -> (.not. x?=w636:bool)
            n83 = Not Equal?(x=w638, y=w642) -> (x != y?=w637:bool)
            n84 = Equal To 0?(x=w638) -> (x = 0?=w640:bool)
            n85 = And(x=w636, y=w640) -> (x .and. y?=w639:bool)
            n86 = case shown="True" w639 {
              tunnel: w638 -> [w646 _]
              tunnel: w637 -> [w645 _]
              tunnel: w636 -> [w644 _]
              frame False {
                n87 = And(x=w644, y=w645) -> (x .and. y?=w643:bool)
                n88 = case shown="False" w643 {
                  tunnel: w646 -> [_ w647]
                  frame False {
                  }
                  frame True {
                    n89 = property on="New: Width" class="DigNum (strict)"("Val(Sgnl)"=w647) -> ()  [unwired: 2 in, 2 out]
                  }
                }
              }
              frame True {
                n90 = local read "Rec: Width"() -> (w648:dbl)
                n91 = local write "New: Width"(w648) -> ()
              }
            }
          }
          frame #2 {
            n92 = local read "Rec: Length"() -> (w655:dbl)
            n93 = case shown="True" w651 {
              frame False {
                n94 = property on="Comments:" class="Str"("DisabledEnum"=T14."Disabled" ("Disabled")) -> ()  [unwired: 2 in, 2 out]
              }
              frame True {
                n95 = property on="Comments:" class="Str"("DisabledEnum"=T14."Enabled" ("Disabled")) -> ()  [unwired: 2 in, 2 out]
              }
            }
            n96 = case shown="False" w654 {
              tunnel: w655 -> [w662 _]
              frame False {
                n97 = local write "New: Length"(w662) -> ()
                n98 = property on="New: Length" class="DigNum (strict)"("DisabledEnum"=T14."Disabled" ("Disabled")) -> ()  [unwired: 2 in, 2 out]
              }
              frame True {
                n99 = property on="New: Length" class="DigNum (strict)"("DisabledEnum"=T14."Enabled" ("Disabled")) -> ()  [unwired: 2 in, 2 out]
              }
            }
            n100 = local read "Rec: Dielectric (d)"() -> (w653:dbl)
            n101 = case shown="True" w652 {
              tunnel: w653 -> [w659 _]
              frame False {
                n102 = local write "New: Dielectric"(w659) -> ()
                n103 = property on="New: Dielectric" class="DigNum (strict)"("DisabledEnum"=T14."Disabled" ("Disabled")) -> ()  [unwired: 2 in, 2 out]
              }
              frame True {
                n104 = property on="New: Dielectric" class="DigNum (strict)"("DisabledEnum"=T14."Enabled" ("Disabled")) -> ()  [unwired: 2 in, 2 out]
              }
            }
          }
        }
        n105 = Strip Path(path=w102) -> (stripped path=w106:path)  [unwired: 1 out]
        n106 = call <vilib>:"Intialize Keyboard.vi"() -> ("device ID"=w150:refnum<k1>)  [unwired: 10 in, 1 out]
        n107 = Subtract(x=w109, y=w162) -> (x-y=w117:sgl)
        n108 = Equal?(x=w127, y=w126) -> (x = y?=w125:bool)
        n109 = List Folder(path=w106) -> (filenames=w105:string[])  [unwired: 3 in, 3 out]
        n110 = call-poly <vilib>:"Acquire Input Data.vi"("device ID"=w150) -> ("keys pressed"=w151:T16)  [unwired: 16 in, 2 out]
        n111 = Unbundle(w130) -> ("X"=w129:i32)  [unwired: 1 out]
        n112 = Reciprocal(x=w173) -> (1/x=w174:sgl)
        n113 = Index Array(array=w151) -> (element=w111:T17)  [unwired: 1 in]
        n114 = Array Size(array=w105) -> (size(s)=w101:i32)
        n115 = To Single Precision Float(number=w107) -> (single precision float=w108:sgl)
        n116 = To Single Precision Float(number=w109) -> (single precision float=w110:sgl)
        n117 = local write "Zoom"(w129) -> ()
        n118 = Multiply(x=w174, y=sgl 50.0) -> (x*y=w172:sgl)
        n119 = property on="Next File" class="Bool (strict)"("Value"=w177) -> (error out=w183:errorcluster)  [unwired: 2 in, 1 out]
        n120 = Add(x=w117, y=w164) -> (x+y=w115:sgl)
        n121 = Subtract(x=w107, y=w163) -> (x-y=w119:sgl)
        n122 = Add(x=w119, y=w165) -> (x+y=w113:sgl)
        n123 = case shown="\"UP\"" w111 {
          tunnel: w110 -> [w232 w238 w242 w244 w248 w250 w252 w254 w256 w258 w260 w262 w264 w266 w268 w270 w272 w274 w276 w278 w280 w282 w284 w286 w288 w290 w292 w294 w296 w298 w300 w302 w304 w306 w308 w310 w312 w314 w316 w318 w320 w322 w324 w326 w328 w330 w332 w334 w336 w338 w340 w342 w344 w346 w348 w350 w352 w354 w356 w358 w360 w362 w364 w366 w368 w370 w372 w374 w376 w378 w380 w382 w384 w386 w388 w390 w392 w394 w396 w398 w400 w402 w404 w406 w408 w410 w412 w414 w416 w418 w420 w422 w424 w426 w428 w430 w432 w434 w436 w438 w440 w442 w444 w446 w448]
          tunnel: [w232 w237 w241 w244 w248 w250 w252 w254 w256 w258 w260 w262 w264 w266 w268 w270 w272 w274 w276 w278 w280 w282 w284 w286 w288 w290 w292 w294 w296 w298 w300 w302 w304 w306 w308 w310 w312 w314 w316 w318 w320 w322 w324 w326 w328 w330 w332 w334 w336 w338 w340 w342 w344 w346 w348 w350 w352 w354 w356 w358 w360 w362 w364 w366 w368 w370 w372 w374 w376 w378 w380 w382 w384 w386 w388 w390 w392 w394 w396 w398 w400 w402 w404 w406 w408 w410 w412 w414 w416 w418 w420 w422 w424 w426 w428 w430 w432 w434 w436 w438 w440 w442 w444 w446 w448] -> w148
          tunnel: w108 -> [w234 w236 w240 w246 w247 w249 w251 w253 w255 w257 w259 w261 w263 w265 w267 w269 w271 w273 w275 w277 w279 w281 w283 w285 w287 w289 w291 w293 w295 w297 w299 w301 w303 w305 w307 w309 w311 w313 w315 w317 w319 w321 w323 w325 w327 w329 w331 w333 w335 w337 w339 w341 w343 w345 w347 w349 w351 w353 w355 w357 w359 w361 w363 w365 w367 w369 w371 w373 w375 w377 w379 w381 w383 w385 w387 w389 w391 w393 w395 w397 w399 w401 w403 w405 w407 w409 w411 w413 w415 w417 w419 w421 w423 w425 w427 w429 w431 w433 w435 w437 w439 w441 w443 w445 w447]
          tunnel: [w233 w236 w240 w245 w247 w249 w251 w253 w255 w257 w259 w261 w263 w265 w267 w269 w271 w273 w275 w277 w279 w281 w283 w285 w287 w289 w291 w293 w295 w297 w299 w301 w303 w305 w307 w309 w311 w313 w315 w317 w319 w321 w323 w325 w327 w329 w331 w333 w335 w337 w339 w341 w343 w345 w347 w349 w351 w353 w355 w357 w359 w361 w363 w365 w367 w369 w371 w373 w375 w377 w379 w381 w383 w385 w387 w389 w391 w393 w395 w397 w399 w401 w403 w405 w407 w409 w411 w413 w415 w417 w419 w421 w423 w425 w427 w429 w431 w433 w435 w437 w439 w441 w443 w445 w447] -> w149
          tunnel: w172 -> [w231 w235 w239 w243 _ _ _ _ _ _ _ _ _ _ _ _ _ _ _ _ _ _ _ _ _ _ _ _ _ _ _ _ _ _ _ _ _ _ _ _ _ _ _ _ _ _ _ _ _ _ _ _ _ _ _ _ _ _ _ _ _ _ _ _ _ _ _ _ _ _ _ _ _ _ _ _ _ _ _ _ _ _ _ _ _ _ _ _ _ _ _ _ _ _ _ _ _ _ _ _ _ _ _ _ _]
          frame "DOWN" {
            n124 = Add(x=w234, y=w231) -> (x+y=w233:sgl)
          }
          frame "LEFT" {
            n125 = Subtract(x=w238, y=w235) -> (x-y=w237:sgl)
          }
          frame "RIGHT" {
            n126 = Add(x=w242, y=w239) -> (x+y=w241:sgl)
          }
          frame "UP" {
            n127 = Subtract(x=w246, y=w243) -> (x-y=w245:sgl)
          }
          frame "ENTER (num pad)" {
          }
          frame "' (quote)" {
          }
          frame "END" {
          }
          frame "EQUALS" {
          }
          frame "ESCAPE" {
          }
          frame "GRAVE (`)" {
          }
          frame "HOME" {
          }
          frame "INSERT" {
          }
          frame "LBRACKET" {
          }
          frame "LCONTROL" {
          }
          frame "L ALT" {
          }
          frame "LSHIFT" {
          }
          frame "LWIN" {
          }
          frame "MINUS" {
          }
          frame "MULTIPLY" {
          }
          frame "NEXT" {
          }
          frame "NUMLOCK" {
          }
          frame "NUMPAD_0" {
          }
          frame "NUMPAD_1" {
          }
          frame "NUMPAD_2" {
          }
          frame "NUMPAD_3" {
          }
          frame "NUMPAD_4" {
          }
          frame "NUMPAD_5" {
          }
          frame "NUMPAD_6" {
          }
          frame "NUMPAD_7" {
          }
          frame "NUMPAD_8" {
          }
          frame "NUMPAD_9" {
          }
          frame "PAUSE" {
          }
          frame "PERIOD" {
          }
          frame "PRIOR (PG UP)" {
          }
          frame "RBRACKET" {
          }
          frame "RCONTROL" {
          }
          frame "RETURN" {
          }
          frame "R ALT" {
          }
          frame "RSHIFT" {
          }
          frame "RWIN" {
          }
          frame "SCROLL" {
          }
          frame "SEMICOLON" {
          }
          frame "SLASH" {
          }
          frame "SPACE" {
          }
          frame "SUBTRACT" {
          }
          frame "TAB" {
          }
          frame "DIVIDE" {
          }
          frame "DELETE" {
          }
          frame "DECIMAL" {
          }
          frame "COMMA" {
          }
          frame "CAPITAL" {
          }
          frame "BACKSLASH" {
          }
          frame "BACK" {
          }
          frame "ADD" {
          }
          frame "F15" {
          }
          frame "F14" {
          }
          frame "F13" {
          }
          frame "F12" {
          }
          frame "F11" {
          }
          frame "F10" {
          }
          frame "F9" {
          }
          frame "F8" {
          }
          frame "F7" {
          }
          frame "F6" {
          }
          frame "F5" {
          }
          frame "F4" {
          }
          frame "F3" {
          }
          frame "F2" {
          }
          frame "F1" {
          }
          frame "Z" {
          }
          frame "Y" {
          }
          frame "X" {
          }
          frame "W" {
          }
          frame "V" {
          }
          frame "U" {
          }
          frame "T" {
          }
          frame "S" {
          }
          frame "R" {
          }
          frame "Q" {
          }
          frame "P" {
          }
          frame "O" {
          }
          frame "N" {
          }
          frame "M" {
          }
          frame "L" {
          }
          frame "K" {
          }
          frame "J" {
          }
          frame "I" {
          }
          frame "H" {
          }
          frame "G" {
          }
          frame "F" {
          }
          frame "E" {
          }
          frame "D" {
          }
          frame "C" {
          }
          frame "B" {
          }
          frame "A" {
          }
          frame "9" {
          }
          frame "8" {
          }
          frame "7" {
          }
          frame "6" {
          }
          frame "5" {
          }
          frame "4" {
          }
          frame "3" {
          }
          frame "2" {
          }
          frame "1" {
          }
          frame "0" {
          }
        }
        n128 = To Long Integer(number=w117) -> (32bit integer=w116:i32)
        n129 = To Long Integer(number=w113) -> (32bit integer=w112:i32)
        n130 = To Long Integer(number=w115) -> (32bit integer=w114:i32)
        n131 = case shown="True" w125 {
          tunnel: w109 -> [w195 _]
          frame False {
            n132 = local write "Image Center X"(w195) -> ()
          }
          frame True {
          }
        }
        n133 = To Long Integer(number=w119) -> (32bit integer=w118:i32)
        n134 = Divide(x=w99, y=w101) -> (x/y=w100:dbl)
        n135 = property on="Previous File" class="Bool (strict)"(error in=w183, "Value"=w177) -> (error out=w182:errorcluster)  [unwired: 1 in, 1 out]
        n136 = Divide(x=sgl 20.0, y=w173) -> (x/y=w171:sgl)
        n137 = Bundle(w148, w149) -> (w122:cluster{sgl, sgl})  [unwired: 1 in]
        n138 = Bundle(w116, w118, w114, w112, 0.0) -> (w120:cluster{i32, i32, i32, i32, dbl})  [unwired: 1 in]
        n139 = Multiply(x=w100, y=100) -> (x*y=→"Progress":dbl)
        n140 = To Unsigned Long Integer(number=w122) -> (unsigned 32bit integer=w121:cluster{u32, u32})
        n141 = property on="Save" class="Bool (strict)"(error in=w182, "Value"=w177) -> (error out=w181:errorcluster)  [unwired: 1 in, 1 out]
        n142 = property on="Export" class="Bool (strict)"("Value"=w177) -> ()  [unwired: 2 in, 2 out]
        n143 = call "IMAQ Convert Rectangle to ROI (Polygon)"("Rectangle"=w120) -> ("ROI Descriptor"=w154:T18)  [unwired: 7 in, 2 out]
        n144 = property on="Save Next" class="Bool (strict)"(error in=w181, "Value"=w177) -> (error out=w180:errorcluster)  [unwired: 1 in, 1 out]
        n145 = property on="Discard" class="Bool (strict)"(error in=w180, "Value"=w177) -> (error out=w179:errorcluster)  [unwired: 1 in, 1 out]
        n146 = property on="Save Lines" class="Bool (strict)"(error in=w179, "Value"=w177) -> ()  [unwired: 1 in, 2 out]
        n147 = property on="Image Preview" class="ImageControl"("ROI"=w154) -> ()  [unwired: 2 in, 2 out]
        n148 = property on="Close" class="Bool (strict)"("Value"=w177) -> ()  [unwired: 2 in, 2 out]
        n149 = Bundle("Application Font", w171, w167, w167, w167, w167, w167, TRUE, w169) -> (w166:T19)  [unwired: 1 in]
        n150 = property on="Image Out" class="ImageControl"("Image Center Position"=w121) -> ()  [unwired: 2 in, 2 out]
        n151 = property on="Disable Flag" class="Bool (strict)"("Value"=w177) -> ()  [unwired: 2 in, 2 out]
        n152 = Bundle(w169, w166, w169, w169) -> (w132:T20)  [unwired: 1 in]
        n153 = Cluster To Array(cluster=w176) -> (array=w193:bool[])
        n154 = local read "Image Out"() -> (w131:T9)
        n155 = property on="Image Out" class="ImageControl"() -> ("ROI"=w134:T21)  [unwired: 2 in, 2 out]
        n156 = Unbundle By Name(w134) -> ("Contours"=w135:T22)
        n157 = local read "Scale Factors"() -> (w98:T11)
        n158 = call "IMAQ Clear Overlay"("Image"=w131) -> ("Image Out"=w147:T9)  [unwired: 9 in, 1 out]
        n159 = Initialize Array(0) -> (w137:i32[])  [unwired: 1 in]
        n160 = Array Size(array=w135) -> (size(s)=w136:i32)
        n161 = Cluster To Array(cluster=w98) -> (array=w97:dbl[])
        n162 = call "Next State.vi"("Buttons []"=w193, "States []"=w194) -> ("Enum"=w186:T2)  [unwired: 1 out]
        n163 = event shown="[8] \"Sat-Log Slider\": Value Change" {
          selector: _ -> [_ _ _ _ _ _ _ _ _ _ _ _ _ _ _ _ _ _ _]
          dyn-events: _ -> [_ _ _ _ _ _ _ _ _ _ _ _ _ _ _ _ _ _ _]
          timeout: 50 -> [_ _ _ _ _ _ _ _ _ _ _ _ _ _ _ _ _ _ _]
          tunnel: w186 -> [w450 _ _ _ _ _ _ _ _ _ _ _ _ _ _ _ _ _ _]
          tunnel: [w450 MegaAwesome_States."Re-Calculated Values" MegaAwesome_States."Calculated Values" MegaAwesome_States."Calculated Values" MegaAwesome_States."Calculated Values" MegaAwesome_States."Calculated Values" MegaAwesome_States."Re-Calculated Values" MegaAwesome_States."Re-Calculated Values" MegaAwesome_States."Re-Calculated Values" MegaAwesome_States."Save" MegaAwesome_States."Re-Calculated Values" MegaAwesome_States."Read Data" MegaAwesome_States."Read Data" MegaAwesome_States."No Event" MegaAwesome_States."No Event" MegaAwesome_States."No Event" MegaAwesome_States."No Event" MegaAwesome_States."No Event" MegaAwesome_States."No Event"] -> w185
          tunnel: w99 -> [w449 w451 w453 w455 w457 w459 w474 w501 w535 w559 w565 _ w592 w594 w607 w609 w613 w617 w621]
          tunnel: [w449 w451 w453 w455 w457 w459 w474 w501 w535 w559 w565 w582 w592 w594 w607 w609 w613 w617 w621] -> w178
          tunnel: w96 -> [_ _ _ _ _ _ _ _ _ _ _ w581 _ _ _ _ _ _ _]
          tunnel: w176 -> [_ _ _ _ _ _ _ _ _ _ _ _ _ _ _ _ _ _ _]
          event Timeout {
            n164 = event-data() -> ()  [unwired: 1 in, 2 out]
          }
          event "New: Dielectric", "New: Width", "New: Length", "New: Temp": Value Change {
            n165 = event-data() -> ()  [unwired: 1 in, 5 out]
          }
          event "Num Pts Log", "Transport Style Controls", "Num Pts": Value Change {
            n166 = event-data() -> ()  [unwired: 1 in, 5 out]
          }
          event "Dielectric Constant": Value Change {
            n167 = event-data() -> ()  [unwired: 1 in, 5 out]
          }
          event "Vd_Lin Index": Value Change {
            n168 = event-data() -> ()  [unwired: 1 in, 5 out]
          }
          event "Vd_Sat Index": Value Change {
            n169 = event-data() -> ()  [unwired: 1 in, 5 out]
          }
          event "Sat-Trans Slider": Value Change {
            n170 = event-data() -> ()  [unwired: 1 in, 5 out]
            n171 = local read "Hysteresis Analysis"() -> (w468:enum32{"1st Sweep", "2nd Sweep", "Both"})
            n172 = local read "Sqrt-Sat"() -> (w462:cluster{dbl[], dbl[]}[])
            n173 = Index Array(array=w462) -> (element=w467:cluster{dbl[], dbl[]})  [unwired: 1 in]
            n174 = Index Array(array=w462, index=1) -> (element=w466:cluster{dbl[], dbl[]})
            n175 = Index Array(array=w462, index=2) -> (element=w461:cluster{dbl[], dbl[]})
            n176 = case shown="\"Both\"" w468 {
              tunnel: w467 -> [w487 _ w497]
              tunnel: [w487 w488 w489] -> w465
              tunnel: w466 -> [_ w488 w496]
              frame "1st Sweep", Default {
              }
              frame "2nd Sweep" {
              }
              frame "Both" {
                n177 = Unbundle(w497) -> (w495:dbl[], w493:dbl[])
                n178 = Unbundle(w496) -> (w494:dbl[], w492:dbl[])
                n179 = Insert Into Array(array=w495, new element=w494) -> (w491:dbl[])  [unwired: 1 in]
                n180 = Insert Into Array(array=w493, new element=w492) -> (w490:dbl[])  [unwired: 1 in]
                n181 = Bundle(w491, w490) -> (w489:cluster{dbl[], dbl[]})  [unwired: 1 in]
              }
            }
            n182 = local read "Sat-Trans Slider"() -> (w472:dbl)
            n183 = local read "Num Pts"() -> (w475:i32)
            n184 = Unbundle(w465) -> (w470:dbl[], w473:dbl[])
            n185 = local read "New: Dielectric"() -> (w484:dbl)
            n186 = local read "New: Width"() -> (w486:dbl)
            n187 = local read "New: Length"() -> (w485:dbl)
            n188 = Array Subset(array=w470, index=w472, length=w475) -> (w482:dbl[])
            n189 = Array Subset(array=w473, index=w472, length=w475) -> (w483:dbl[])
            n190 = Index Array(array=w470, index=w472) -> (element=w471:dbl)
            n191 = call "Mobility-Vt-Used Pts_Saturation.vi"("Width"=w486, "Length"=w485, "Dielectric (d)"=w484, "Sat Id Used"=w483, "Vg Used"=w482) -> ("Vt"=w478:dbl, "Mobility"=w479:dbl)  [unwired: 4 in, 1 out]
            n192 = local write "Index-Sat"(w472) -> ()
            n193 = local write "Sat Id-Used"(w483) -> ()
            n194 = Bundle(w482, w483) -> (w464:cluster{dbl[], dbl[]})  [unwired: 1 in]
            n195 = local read "Re-Calculated Values Cluster"() -> (w481:T10)
            n196 = Bundle By Name(cluster=w481, "Mobility-Sat"=w479, "Vt-Sat"=w478) -> (w480:T10)
            n197 = local write "Re-Calculated Values Cluster"(w480) -> ()
            n198 = local write "Sat Vg Array-Used"(w482) -> ()
            n199 = local write "Used Vg \nSqrt Sat"(w471) -> ()
            n200 = Build Array(w467, w466, w461, w464) -> (w476:cluster{dbl[], dbl[]}[])
            n201 = local write "Sqrt-Sat"(w476) -> ()
          }
          event "Lin-Trans Slider": Value Change {
            n202 = event-data() -> ()  [unwired: 1 in, 5 out]
            n203 = local read "Sqrt-Lin"() -> (w520:cluster{dbl[], dbl[]}[])
            n204 = Decimate 1D Array(w520) -> (w505:cluster{dbl[], dbl[]}[], w506:cluster{dbl[], dbl[]}[])
            n205 = Array To Cluster(array=w505) -> (cluster=w519:T23)
            n206 = local read "Lin-Trans Slider"() -> (w499:dbl)
            n207 = local read "New: Dielectric"() -> (w513:dbl)
            n208 = local read "Num Pts"() -> (w516:i32)
            n209 = local read "New: Width"() -> (w515:dbl)
            n210 = local read "New: Length"() -> (w514:dbl)
            n211 = local read "Lin Vd"() -> (w502:dbl)
            n212 = Unbundle(w519) -> ("[0]"=w518:cluster{dbl[], dbl[]})  [unwired: 8 out]
            n213 = Unbundle(w518) -> (w500:dbl[], w517:dbl[])
            n214 = Search 1D Array(1D array=w500, element=w499) -> (index of element=w498:i32)  [unwired: 1 in]
            n215 = Array Subset(array=w500, index=w498, length=w516) -> (w511:dbl[])
            n216 = local write "Lin-Vg Array-Used"(w511) -> ()
            n217 = Array Subset(array=w517, index=w498, length=w516) -> (w512:dbl[])
            n218 = call "Mobility-Vt-Used Pts_Linear.vi"("Width"=w515, "Length"=w514, "Vd"=w502, "Dielectric (d)"=w513, "Id Used"=w512, "Vg Used"=w511) -> ("Mobility"=w508:dbl)  [unwired: 3 in, 2 out]
            n219 = local write "Index-Lin"(w498) -> ()
            n220 = local write "Lin Id-Used"(w512) -> ()
            n221 = Bundle(w511, w512) -> (w507:cluster{dbl[], dbl[]})  [unwired: 1 in]
            n222 = local read "Re-Calculated Values Cluster"() -> (w510:T10)
            n223 = Bundle By Name(cluster=w510, "Moblitity-Lin"=w508) -> (w509:T10)
            n224 = local write "Re-Calculated Values Cluster"(w509) -> ()
            n225 = Build Array (concatenate)(w505, w506, w507) -> (w504:cluster{dbl[], dbl[]}[])
            n226 = local write "Sqrt-Lin"(w504) -> ()
          }
          event "Sat-Log Slider": Value Change {
            n227 = local read "Hysteresis Analysis"() -> (w529:enum32{"1st Sweep", "2nd Sweep", "Both"})
            n228 = event-data() -> ()  [unwired: 1 in, 5 out]
            n229 = disable-structure shown="Disabled" {
              frame Disabled {
                n230 = property on="Sat-Log" class="XYGraph (strict)"("Active Plot"=u32 2, "Plot.Fill/Pt. Color"=u32 6618880, "Plot.Point Style"=u8 11) -> ()  [unwired: 2 in, 2 out]
              }
              frame Enabled {
              }
            }
            n231 = local read "Sat-Log"() -> (w526:cluster{dbl[], dbl[]}[])
            n232 = local read "Num Pts Log"() -> (w543:i32)
            n233 = local read "Sat-Log Slider"() -> (w530:dbl)
            n234 = Index Array(array=w526) -> (element=w523:cluster{dbl[], dbl[]})  [unwired: 1 in]
            n235 = Index Array(array=w526, index=1) -> (element=w522:cluster{dbl[], dbl[]})
            n236 = case shown="\"2nd Sweep\"" w529 {
              tunnel: w523 -> [w548 _ w558]
              tunnel: [w548 w549 w550] -> w521
              tunnel: w522 -> [_ w549 w557]
              frame "1st Sweep", Default {
              }
              frame "2nd Sweep" {
              }
              frame "Both" {
                n237 = Unbundle(w558) -> (w556:dbl[], w554:dbl[])
                n238 = Unbundle(w557) -> (w555:dbl[], w553:dbl[])
                n239 = Insert Into Array(array=w556, new element=w555) -> (w552:dbl[])  [unwired: 1 in]
                n240 = Insert Into Array(array=w554, new element=w553) -> (w551:dbl[])  [unwired: 1 in]
                n241 = Bundle(w552, w551) -> (w550:cluster{dbl[], dbl[]})  [unwired: 1 in]
              }
            }
            n242 = Index Array(array=w526, index=2) -> (element=w524:cluster{dbl[], dbl[]})
            n243 = Unbundle(w521) -> (w531:dbl[], w544:dbl[])
            n244 = Array Subset(array=w531, index=w530, length=w543) -> (w541:dbl[])
            n245 = To Single Precision Float(number=w530) -> (single precision float=w533:sgl)
            n246 = To Single Precision Float(number=w531) -> (single precision float=w534:sgl[])
            n247 = Search 1D Array(1D array=w534, element=w533) -> ()  [unwired: 1 in, 1 out]
            n248 = Array Subset(array=w544, index=w530, length=w543) -> (w542:dbl[])
            n249 = local write "Vg Array-Log-Used"(w541) -> ()
            n250 = local write "IndexLog-Sat"(w530) -> ()
            n251 = Bundle(w541, w542) -> (w525:cluster{dbl[], dbl[]})  [unwired: 1 in]
            n252 = call "STS-Used.vi"("Id Used"=w542, "Vg-Used"=w541) -> ("STS"=w538:dbl)  [unwired: 9 in]
            n253 = local write "Sat Id-Log-Used"(w542) -> ()
            n254 = Index Array(array=w531, index=w530) -> (element=w532:dbl)
            n255 = local read "Re-Calculated Values Cluster"() -> (w540:T10)
            n256 = Bundle By Name(cluster=w540, "STS"=w538) -> (w539:T10)
            n257 = local write "Re-Calculated Values Cluster"(w539) -> ()
            n258 = local write "Used Vg \nLog Sat"(w532) -> ()
            n259 = Build Array(w523, w522, w524, w525) -> (w537:cluster{dbl[], dbl[]}[])
            n260 = local write "Sat-Log"(w537) -> ()
          }
          event "File Controls.Save Next": Mouse Down {
            n261 = event-data() -> ()  [unwired: 1 in, 5 out]
            "Save Next?" <- TRUE ("Save Next?")
          }
          event "Lin-Log Slider": Value Change {
            n262 = event-data() -> ()  [unwired: 1 in, 5 out]
            n263 = local read "Lin-Log"() -> (w568:cluster{dbl[], dbl[]}[])
            n264 = Decimate 1D Array(w568) -> (w570:cluster{dbl[], dbl[]}[], w571:cluster{dbl[], dbl[]}[])
            n265 = disable-structure shown="Disabled" {
              frame Disabled {
                n266 = property on="Lin-Log" class="XYGraph (strict)"("Active Plot"=u32 2, "Plot.Fill/Pt. Color"=u32 6618880, "Plot.Point Style"=u8 11) -> ()  [unwired: 2 in, 2 out]
              }
              frame Enabled {
              }
            }
            n267 = Array To Cluster(array=w570) -> (cluster=w577:T23)
            n268 = local read "Num Pts Log"() -> (w574:i32)
            n269 = local read "Lin-Log Slider"() -> (w562:dbl)
            n270 = Unbundle(w577) -> ("[0]"=w576:cluster{dbl[], dbl[]})  [unwired: 8 out]
            n271 = Unbundle(w576) -> (w563:dbl[], w575:dbl[])
            n272 = Index Array(array=w563, index=w562) -> (element=w564:dbl)
            n273 = local write "Used Vg \nLog Lin"(w564) -> ()
            n274 = Search 1D Array(1D array=w563, element=w562) -> ()  [unwired: 1 in, 1 out]
            n275 = Array Subset(array=w563, index=w562, length=w574) -> (w572:dbl[])
            n276 = local write "Lin-Vg Array-Log Used"(w572) -> ()
            n277 = Array Subset(array=w575, index=w562, length=w574) -> (w573:dbl[])
            n278 = local write "IndexLog-Sat"(w562) -> ()
            n279 = Bundle(w572, w573) -> (w567:cluster{dbl[], dbl[]})  [unwired: 1 in]
            n280 = local write "Lin Id-Log Used"(w573) -> ()
            n281 = Build Array (concatenate)(w570, w571, w567) -> (w569:cluster{dbl[], dbl[]}[])
            n282 = local write "Lin-Log"(w569) -> ()
          }
          event "Index Array": Value Change {
            n283 = event-data() -> ()  [unwired: 1 in, 5 out]
            n284 = Strip Path(path=w581) -> (stripped path=w587:path)  [unwired: 1 out]
            n285 = local write "Transfer Folder"(w587) -> ()
            n286 = List Folder(path=w587) -> (filenames=w583:string[])  [unwired: 3 in, 3 out]
            n287 = local read "Index Array"() -> (w582:i32)
            n288 = Path To String(path=w587) -> (string=w588:string)
            n289 = Index Array(array=w583, index=w582) -> (element=w589:string)
            n290 = Concatenate Strings(w588, "\\", w589) -> (w585:string)
            n291 = String To Path(string=w585) -> (path=w584:path)
            n292 = local write "Transfer File"(w584) -> ()
          }
          event "Transfer File": Value Change {
            w591 = path ""
            n293 = event-data() -> ()  [unwired: 1 in, 5 out]
            n294 = local write "Transport\nFolder"(w591) -> ()
            n295 = local write "Image Folder"(w591) -> ()
          }
          event "Remove Button": Mouse Down {
            w596 = 0
            n296 = event-data() -> ()  [unwired: 1 in, 5 out]
            n297 = property on="Image Out" class="ImageControl"() -> ("ROI"=w606:T21)  [unwired: 2 in, 2 out]
            n298 = Unbundle(w606) -> ("Global Rectangle"=w597:i32[], "Contours"=w599:T22)
            n299 = Reverse 1D Array(array=w597) -> (reversed array=w598:i32[])
            n300 = Reverse 1D Array(array=w599) -> (reversed array=w600:T22)
            n301 = Delete From Array(array=w598, index=w596) -> (array with subset deleted=w601:i32[])  [unwired: 1 in, 1 out]
            n302 = Delete From Array(array=w600, index=w596) -> (array with subset deleted=w602:T22)  [unwired: 1 in, 1 out]
            n303 = Reverse 1D Array(array=w601) -> (reversed array=w603:i32[])
            n304 = Reverse 1D Array(array=w602) -> (reversed array=w604:T22)
            n305 = Bundle(w603, w604) -> (w605:T24)  [unwired: 1 in]
            n306 = property on="Image Out" class="ImageControl"("ROI"=w605) -> ()  [unwired: 2 in, 2 out]
          }
          event "Undo Button": Mouse Down {
            n307 = event-data() -> ()  [unwired: 1 in, 5 out]
            n308 = invoke on="Image Out" class="ImageControl" method="Clear ROI"() -> ()  [unwired: 3 in, 3 out]
          }
          event "Image Folder": Value Change {
            n309 = event-data() -> ()  [unwired: 1 in, 5 out]
            n310 = local read "Image File"() -> (w611:path)
            n311 = call "Vision Acquisition"("Image Path"=w611) -> ("Image Out"=w612:T9)  [unwired: 25 in, 1 out]
            n312 = local write "Image Preview"(w612) -> ()
            n313 = local write "Image Out"(w612) -> ()
          }
          event "Zoom": Value Change {
            n314 = event-data() -> ()  [unwired: 1 in, 5 out]
            n315 = local read "Zoom"() -> (w616:i32)
            n316 = Bundle("Zoom"=w616, "Zoom"=w616) -> (w615:cluster{"Zoom":i32, "Zoom":i32})  [unwired: 1 in]
            n317 = property on="Image Out" class="ImageControl"("ZoomInteger"=w615) -> ()  [unwired: 2 in, 2 out]
          }
          event "Image Out": Mouse Enter {
            n318 = event-data() -> ()  [unwired: 1 in, 3 out]
            n319 = call "Simulate_Keyboard.vi"("Action"=u32 0, "Virtual Key"=u8 162) -> ()  [unwired: 7 in, 1 out]
          }
          event "Image Out": Mouse Leave {
            n320 = event-data() -> ()  [unwired: 1 in, 3 out]
            n321 = flat-sequence {
              frame #0 {
                n322 = Wait (ms)(milliseconds to wait=u32 10) -> ()  [unwired: 1 out]
              }
              frame #1 {
                n323 = call "Simulate_Keyboard.vi"("Action"=u32 2, "Virtual Key"=u8 162) -> ()  [unwired: 7 in, 1 out]
              }
            }
          }
        }
        n324 = Build Array(0.5495, 0.2755, 0.1389, 0.0546, 0.0337) -> ()  [unwired: 1 out]
        n325 = Array Subset(array=w97, index="Magnification", length=1) -> (w145:dbl[])
        n326 = To Double Precision Float(number=w145) -> (double precision float=w146:dbl[])
        n327 = for {
          N: w136 -> [_]
          shift-right: [w221] -> _
          shift-left: w135 -> [w221]
          shift-right: [w198] -> w123
          shift-left: w137 -> [w219]
          tunnel: w146 -> [w218]
          shift-right: [w215] -> _
          shift-left: w147 -> [w217]
          tunnel: w132 -> [w211]
          i -> [w214]
          n328 = Index Array(array=w221, index=w214) -> (element=w230:T25)
          n329 = Unbundle(w230) -> ("Points"=w229:i32[])  [unwired: 2 out]
          n330 = Array To Cluster(array=w229) -> (cluster=w228:T26)
          n331 = Unbundle(w228) -> ("Points[0]"=w210:i32, "Points[1]"=w197:i32, "Points[2]"=w220:i32, "Points[3]"=w226:i32)  [unwired: 5 out]
          n332 = Add(x=w210, y=10) -> (x+y=w208:i32)
          n333 = Subtract(x=w197, y=w226) -> (x-y=w225:i32)
          n334 = Subtract(x=w210, y=w220) -> (x-y=w227:i32)
          n335 = Square(x=w225) -> (x^2=w223:i32)
          n336 = Square(x=w227) -> (x^2=w224:i32)
          n337 = To Double Precision Float(number=w197) -> (double precision float=w196:dbl)
          n338 = Add(x=w224, y=w223) -> (x+y=w222:i32)
          n339 = Square Root(x=w222) -> (sqrt(x)=w202:dbl)
          n340 = Multiply(x=w202, y=0.5) -> (x*y=w205:dbl)
          n341 = Multiply(x=w202, y=w218) -> (x*y=w201:dbl[])
          n342 = Index Array(array=w201) -> (element=w213:dbl)  [unwired: 1 in]
          n343 = Number To Fractional String(number=w213, precision (6)=0) -> (F-format string=w212:string)  [unwired: 2 in]
          n344 = Build Array (concatenate)(w219, w201) -> (w199:dbl[])
          n345 = Add(x=w205, y=w196) -> (x+y=w207:dbl)
          n346 = Bundle(w208, w207) -> (w216:cluster{i32, dbl})  [unwired: 1 in]
          n347 = call "IMAQ Overlay Text"("BG Color (Transparent)"=u32 0, "Text Color (black)"=u32 16448250, "Font, Size & Style"=w211, "String"=w212, "Origin"=w216, "Image"=w217) -> ("Image Out"=w215:T9)  [unwired: 4 in, 1 out]
          n348 = To Long Integer(number=w199) -> (32bit integer=w198:i32[])
        }
        "Distances" <- w123
        n349 = Add Array Elements(numeric array=w123) -> (sum=w133:i32)
        n350 = local write "Total Width"(w133) -> ()
      }
      frame "Read Data" {
        n351 = call "IMAQ Dispose"("All Images? (No)"=TRUE) -> ()  [unwired: 5 in, 1 out]
        n352 = case shown="True" "Disable Flag 2" {
          tunnel: w676 -> [_ w708]
          tunnel: [w704 w705] -> _
          tunnel: w675 -> [w704 _]
          frame False {
          }
          frame True {
            n353 = local read "Transfer Folder"() -> (w707:path)
            n354 = List Folder(path=w707) -> (filenames=w709:string[])  [unwired: 3 in, 3 out]
            n355 = Index Array(array=w709, index=w708) -> (element=w706:string)
            n356 = Build Path(base path=w707, name or relative path=w706) -> (appended path=w705:path)
            n357 = local write "Transfer File"(w705) -> ()
          }
        }
        n358 = case shown="True" "Disable Flag" {
          tunnel: w676 -> [_ w714]
          tunnel: [w710 w711] -> w685
          tunnel: w683 -> [w710 _]
          frame False {
          }
          frame True {
            n359 = local read "Transfer Folder"() -> (w713:path)
            n360 = List Folder(path=w713) -> (filenames=w715:string[])  [unwired: 3 in, 3 out]
            n361 = Index Array(array=w715, index=w714) -> (element=w712:string)
            n362 = Build Path(base path=w713, name or relative path=w712) -> (appended path=w711:path)
            n363 = local write "Transfer File"(w711) -> ()
          }
        }
        n364 = Unbundle By Name(w674) -> ("Manual-Width"=w673:bool, "Manuel-Length"=w669:bool, "Manuel-Dielectric"=w665:bool)  [unwired: 2 out]
        n365 = local read "New: Length"() -> (w666:dbl)
        n366 = local read "New: Width"() -> (w670:dbl)
        n367 = call "Recorded Values.vi"("Path"=w685) -> ("Recorded Char"=→"Recorded Values Cluster":T10, "Recorded Prop"=w694:T1, "Fabrication Prop"=w692:T4)  [unwired: 8 in]
        n368 = Strip Path(path=w685) -> (stripped path=w691:path, name=w690:string)
        n369 = local write "Recorded Prop"(w694) -> ()
        n370 = Unbundle By Name(w694) -> ("Date Recorded"=→"Date Recorded":string, "Index"=w693:string, "Length"=w668:dbl, "Width"=w671:dbl)  [unwired: 1 out]
        n371 = Unbundle By Name(w694) -> ("Sample Temp"=w696:dbl)
        n372 = List Folder(path=w691) -> (filenames=w688:string[])  [unwired: 3 in, 3 out]
        n373 = local write "Fabrication Prop"(w692) -> ()
        n374 = Unbundle By Name(w692) -> ("Dielectric (nm)"=w664:dbl, "Comments"=w689:string, "Date Created"=→"Date Created":string)
        n375 = Select(t=w666, s=w669, f=w668) -> (s? t:f=w667:dbl)
        n376 = Select(t=w670, s=w673, f=w671) -> (s? t:f=w672:dbl)
        n377 = local write "Index"(w693) -> ()
        n378 = local write "Rec: Length"(w668) -> ()
        n379 = local write "Rec: Width"(w671) -> ()
        n380 = Equal To 0?(x=w696) -> (x = 0?=w699:bool)
        n381 = Number To Decimal String(number=w696) -> (decimal integer string=w700:string)  [unwired: 1 in]
        n382 = local write "Comments:"(w689) -> ()
        n383 = Search 1D Array(1D array=w688, element=w690) -> (index of element=w687:i32)  [unwired: 1 in]
        n384 = Equal?(x="", y=w700) -> (x = y?=w698:bool)
        n385 = Index Array(array=w688, index=w687) -> (element=→"Data Name:":string)
        n386 = local write "New: Width"(w672) -> ()
        n387 = local write "New: Length"(w667) -> ()
        n388 = local write "Index Array"(w687) -> ()
        n389 = Or(x=w699, y=w698) -> (x .or. y?=w697:bool)
        n390 = case shown="True" w697 {
          tunnel: [w716 w717] -> w682
          tunnel: w696 -> [w716 _]
          frame False {
          }
          frame True {
            n391 = local read "Room Temp"() -> (w717:dbl)
          }
        }
        n392 = case shown="False" w665 {
          tunnel: w664 -> [w703 _]
          frame False {
            n393 = local write "Rec: Dielectric (d)"(w703) -> ()
            n394 = local write "New: Dielectric"(w703) -> ()
          }
          frame True {
          }
        }
        n395 = local write "New: Temp"(w682) -> ()
        n396 = Bundle By Name(cluster=w694, "Sample Temp"=w682) -> (w695:T1)
        n397 = local write "Rec: Temp"(w682) -> ()
        n398 = local write "Recorded Prop"(w695) -> ()
      }
      frame "Calculated Values" {
        w722 = 0
        w723 = 1
        n399 = local read "Image Center X"() -> (w748:i32)
        n400 = call "Image from TRF Display.vi"("Image Center X"=w748, "No Image File"=w782, "Image Folder"=w783, "Transfer File"=w746) -> ("Image Preview"=w755:T9, "Image Out"=w756:T9, "Image File"=w757:path, "Image Name"=→"Image Name":string, "ROI File"=w752:path)  [unwired: 3 in]
        n401 = invoke on="Image Out" class="ImageControl" method="Clear ROI"() -> ()  [unwired: 3 in, 3 out]
        n402 = local write "Image File"(w757) -> ()
        n403 = local write "Image Out"(w756) -> ()
        n404 = local write "Image Preview"(w755) -> ()
        n405 = call <vilib>:"Check if File or Folder Exists.vi"("path"=w752) -> ("file or folder exists?"=w753:bool, "dup path"=w754:path)  [unwired: 8 in, 1 out]
        n406 = local read "Hysteresis Analysis"() -> (w719:enum32{"1st Sweep", "2nd Sweep", "Both"})
        n407 = case shown="True" w753 {
          tunnel: w754 -> [_ w807]
          frame False {
          }
          frame True {
            n408 = Read from Text File(file (use dialog)=w807) -> (text=w811:string)  [unwired: 3 in, 3 out]
            n409 = property on="Image Out" class="ImageControl"() -> ("ROI"=w808:T21)  [unwired: 2 in, 2 out]
            n410 = Unflatten From String(type=w808, binary string=w811) -> (value=w809:T21, error out=w810:errorcluster)  [unwired: 3 in, 1 out]
            n411 = property on="Image Out" class="ImageControl"(error in=w810, "ROI"=w809) -> ()  [unwired: 1 in, 2 out]
          }
        }
        n412 = call "TRF to LKG Plot_09_11_13a_JW.vi"("Transport Graph Properties"="LKG Style Controls", "No Transport File"=w744, "LKG Folder"=w745, "Transfer File"=w746) -> ("Transport"=w742:cluster{ext[], ext[]}[], "LKG File"=→"LKG (TRF) File":path, "LKG (TRF) Name"=→"LKG (TRF) Name":string)  [unwired: 5 in]
        "LKG (TSF)" <- w742
        n413 = call "TRF to TSP Plot_05_15_13a_JW.vi"("Transport Graph Properties"="Transport Style Controls", "No Transport File"=w744, "Transport Folder"=w758, "Transfer File"=w746) -> ("Transport"=w762:cluster{ext[], ext[]}[], "Transport File"=→"Transport\nFile":path, "Transport Name"=→"Transport Name:":string)  [unwired: 5 in]
        "Transport" <- w762
        n414 = Array Size(array=w762) -> (size(s)=w761:i32)
        n415 = Array Size(array=w742) -> (size(s)=w741:i32)
        n416 = local read "Image Center X"() -> (w749:i32)
        n417 = local read "Recorded Prop"() -> (w785:T1)
        n418 = for {
          N: w761 -> [_]
          tunnel: "Transport Style Controls" -> [w815]
          i -> [w814]
          n419 = Unbundle By Name(w815) -> ("Transport Line Size"=w812:u16, "Transport Line Color"=w813:u32)
          n420 = property on="Transport" class="XYGraph (strict)"("Active Plot"=w814, "Plot.Plot Color"=w813, "Plot.Line Width"=w812) -> ()  [unwired: 2 in, 2 out]
        }
        n421 = for {
          N: w741 -> [_]
          tunnel: "LKG Style Controls" -> [w806]
          i -> [w805]
          n422 = Unbundle By Name(w806) -> ("Transport Line Size"=w803:u16, "LKG (TRF) Line Color"=w804:u32)
          n423 = property on="LKG (TSF)" class="XYGraph (strict)"("Active Plot"=w805, "Plot.Plot Color"=w804, "Plot.Line Width"=w803) -> ()  [unwired: 2 in, 2 out]
        }
        n424 = local read "Fabrication Prop"() -> (w792:T4)
        n425 = Bundle("Image Center X"=w749, 0) -> (w751:cluster{"Image Center X":i32, i32})  [unwired: 1 in]
        n426 = call "Mobility-Vt Calculator-File.vi"("Vd_Sat Index"=w736, "Vd_Lin Index"=w735, "NumPts"=w787, "Hysteresis Analysis"=w719, "Dielectric Constant In"=w738, "Path"=w746) -> ("Used Points"=w780:T27, "Graph Cluster"=w773:T28, "Vd_Lin"=w764:dbl, "Output"=w800:T29, "Vd_Sat"=w737:dbl)  [unwired: 1 in]
        n427 = call "STS Calculator-File.vi"("Hysteresis Analysis"=w719, "NumPts"=w786, "Vd_Lin Index"=w735, "Vd_Sat Index"=w736, "Path"=w746) -> ("Used Points"=w775:T30, "XY Graph-Sat"=w729:cluster{dbl[], dbl[]}[], "XY Graph-Lin"=w765:cluster{dbl[], dbl[]}[], "Ouput"=w795:cluster{"STS-Sat":dbl, "STS-Lin":dbl})  [unwired: 3 in]
        n428 = property on="Image Out" class="ImageControl"("Image Center Position"=w751) -> ()  [unwired: 2 in, 2 out]
        n429 = local read "Calculated Values Cluster"() -> (w802:T10)
        n430 = Unbundle By Name(w792) -> ("Dielectric (nm)"=w790:dbl)
        n431 = Unbundle By Name(w785) -> ("Sample Temp"=w784:dbl)
        n432 = Unbundle By Name(w800) -> ("Mobility-Sat"=w799:dbl, "Vt-Sat"=w791:dbl, "Mobility-Lin"=w798:dbl, "Off I-Sat"=w797:dbl, "On/Off I-Sat"=w796:dbl)  [unwired: 1 out]
        n433 = local write "Lin Vd"(w764) -> ()
        n434 = Unbundle By Name(w795) -> ("STS-Sat"=w789:dbl)  [unwired: 1 out]
        n435 = local write "Vd_Sat"(w737) -> ()
        n436 = local write "Sat-Log"(w729) -> ()
        n437 = local write "Lin-Log"(w765) -> ()
        n438 = call "Trap Density_VT.vi"("VT"=w791, "Dielectric"=w790) -> ("Trap Density-VT"=w794:dbl)
        n439 = call "Trap Density_STS.vi"("Temp (T) [K]"=w784, "S.T.S. (S)"=w789, "Dielectric"=w790) -> ("Trap Density (N)"=w793:dbl)  [unwired: 8 in]
        n440 = Index Array(array=w729, index=1) -> (element=w728:cluster{dbl[], dbl[]})
        n441 = Bundle By Name(cluster=w802, "Mobility-Sat"=w799, "Moblitity-Lin"=w798, "On/Off"=w796, "Off Current"=w797, "Vt-Sat"=w791, "STS"=w789, "Trap Density-VT"=w794, "Trap Density-STS"=w793) -> (w801:T10)
        n442 = Unbundle By Name(w775) -> ("Sat Vg Used"=w718:dbl[], "Sat Log(Id) Used"=w733:dbl[], "Lin Vg Used"=w774:dbl[], "Lin Log(Id) Used"=w731:dbl[], "STS Index-Sat"=w721:dbl, "STS Index-Lin"=w732:dbl)
        n443 = Unbundle By Name(w780) -> ("Sat Vg Used"=w779:dbl[], "Sat Sqrt(Id) Used"=w778:dbl[], "Lin Vg Used"=w777:dbl[], "Lin Sqrt(Id) Used"=w776:dbl[], "Index-Lin"=w769:dbl, "Index-Sat"=w768:dbl)
        n444 = Unbundle(w728) -> (w726:dbl[])  [unwired: 1 out]
        n445 = Array Max & Min(array=w726) -> (max value=w720:dbl)  [unwired: 3 out]
        n446 = Index Array(array=w726, index=w721) -> ()  [unwired: 1 out]
        n447 = local write "Vg Array-Log-Used"(w718) -> ()
        n448 = local write "Sat Id-Log-Used"(w733) -> ()
        n449 = local write "Lin-Vg Array-Log Used"(w774) -> ()
        n450 = local write "Lin Id-Log Used"(w731) -> ()
        n451 = local write "IndexLog-Sat"(w721) -> ()
        n452 = local write "Calculated Values Cluster"(w801) -> ()
        n453 = local write "Sat Vg Array-Used"(w779) -> ()
        n454 = local write "Sat Id-Used"(w778) -> ()
        n455 = local write "Lin-Vg Array-Used"(w777) -> ()
        n456 = Index Array(array=w726, index=w732) -> (element=w730:dbl)
        n457 = local write "IndexLog-Lin"(w730) -> ()
        n458 = local write "Lin Id-Used"(w776) -> ()
        n459 = local write "Index-Sat"(w768) -> ()
        n460 = local write "Index-Lin"(w769) -> ()
        n461 = local write "Used Vg \nLog Sat"(w720) -> ()
        n462 = local write "Lin-Log Slider"(w730) -> ()
        n463 = local write "Sat-Log Slider"(w721) -> ()
        n464 = local write "Sat-Trans Slider"(w768) -> ()
        n465 = local write "Lin-Trans Slider"(w769) -> ()
        n466 = Unbundle By Name(w773) -> ("Raw Sat"=w767:cluster{dbl[], dbl[]}[], "Sqrt Sat"=w770:cluster{dbl[], dbl[]}[], "Raw Lin"=w772:cluster{dbl[], dbl[]}[], "Sqrt Lin"=w771:cluster{dbl[], dbl[]}[])
        n467 = Index Array(array=w767) -> (element=w766:cluster{dbl[], dbl[]})  [unwired: 1 in]
        n468 = Unbundle(w766) -> (w725:dbl[])  [unwired: 1 out]
        n469 = Array Size(array=w725) -> (size(s)=w734:i32)
        n470 = Decrement(x=w734) -> (x-1=w724:i32)
        n471 = property on="Lin-Trans Slider" class="Slide (strict)"("Scale.Maximum"=w724, "Increment"=w723, "Scale.Minimum"=w722) -> ()  [unwired: 2 in, 2 out]
        n472 = property on="Sat-Log Slider" class="Slide (strict)"("Scale.Maximum"=w724, "Increment"=w723, "Scale.Minimum"=w722) -> ()  [unwired: 2 in, 2 out]
        n473 = property on="Lin-Log Slider" class="Slide (strict)"("Scale.Maximum"=w724, "Increment"=w723, "Scale.Minimum"=w722) -> ()  [unwired: 2 in, 2 out]
        n474 = property on="Sat-Trans Slider" class="Slide (strict)"("Scale.Maximum"=w724, "Increment"=w723, "Scale.Minimum"=w722) -> ()  [unwired: 2 in, 2 out]
        n475 = local write "Raw- Sat"(w767) -> ()
        n476 = local write "Raw- Lin"(w772) -> ()
        n477 = local write "Sqrt-Sat"(w770) -> ()
        n478 = local write "Sqrt-Lin"(w771) -> ()
      }
      frame "Re-Calculated Values" {
        n479 = local read "Vg Array-Log-Used"() -> (w825:dbl[])
        n480 = local read "Sat Vg Array-Used"() -> (w833:dbl[])
        n481 = local read "Lin-Vg Array-Used"() -> (w839:dbl[])
        n482 = local read "Sat Id-Log-Used"() -> (w824:dbl[])
        n483 = local read "New: Dielectric"() -> (w837:dbl)
        n484 = local read "New: Dielectric"() -> (w822:dbl)
        n485 = local read "New: Length"() -> (w836:dbl)
        n486 = local read "New: Length"() -> (w832:dbl)
        n487 = local read "New: Width"() -> (w835:dbl)
        n488 = local read "New: Width"() -> (w831:dbl)
        n489 = local read "Lin Id-Used"() -> (w838:dbl[])
        n490 = local read "Sat Id-Used"() -> (w830:dbl[])
        n491 = local read "Re-Calculated Values Cluster"() -> (w841:T10)
        n492 = local read "New: Dielectric"() -> (w821:dbl)
        n493 = local read "New: Temp"() -> (w820:dbl)
        n494 = local read "Lin Vd"() -> (w817:dbl)
        n495 = call "Mobility-Vt-Used Pts_Saturation.vi"("Width"=w831, "Dielectric Const"=w816, "Length"=w832, "Dielectric (d)"=w822, "Sat Id Used"=w830, "Vg Used"=w833) -> ("Vt"=w828:dbl, "Mobility"=w829:dbl)  [unwired: 3 in, 1 out]
        n496 = call "STS-Used.vi"("Id Used"=w824, "Vg-Used"=w825) -> ("STS"=w823:dbl)  [unwired: 9 in]
        n497 = call "Mobility-Vt-Used Pts_Linear.vi"("Width"=w835, "Dielectric Const"=w816, "Length"=w836, "Vd"=w817, "Dielectric (d)"=w837, "Id Used"=w838, "Vg Used"=w839) -> ("Mobility"=w834:dbl)  [unwired: 2 in, 2 out]
        n498 = call "Trap Density_VT.vi"("VT"=w828, "Dielectric"=w822) -> ("Trap Density-VT"=w827:dbl)
        n499 = call "Trap Density_STS.vi"("Temp (T) [K]"=w820, "S.T.S. (S)"=w823, "Dielectric"=w821) -> ("Trap Density (N)"=w819:dbl)  [unwired: 8 in]
        n500 = Bundle By Name(cluster=w841, "Mobility-Sat"=w829, "Moblitity-Lin"=w834, "Vt-Sat"=w828, "STS"=w823, "Trap Density-VT"=w827, "Trap Density-STS"=w819) -> (w840:T10)
        n501 = local write "Re-Calculated Values Cluster"(w840) -> ()
      }
      frame "Next File" {
        n502 = call "IMAQ Dispose"("All Images? (No)"=TRUE) -> ()  [unwired: 5 in, 1 out]
        n503 = Strip Path(path=w858) -> (stripped path=w849:path, name=w856:string)
        n504 = List Folder(path=w849) -> (filenames=w843:string[])  [unwired: 3 in, 3 out]
        n505 = local write "Transfer Folder"(w849) -> ()
        n506 = Array Size(array=w843) -> (size(s)=w855:i32)
        n507 = Search 1D Array(1D array=w843, element=w856) -> (index of element=w853:i32)  [unwired: 1 in]
        n508 = Decrement(x=w855) -> (x-1=w854:i32)
        n509 = Equal?(x=w854, y=w853) -> (x = y?=w852:bool)
        n510 = case shown="True" w852 {
          tunnel: w845 -> [w860 _]
          tunnel: [w859 0] -> w844
          frame False {
            n511 = Increment(x=w860) -> (x+1=w859:i32)
          }
          frame True {
          }
        }
        n512 = Path To String(path=w849) -> (string=w850:string)
        n513 = Index Array(array=w843, index=w844) -> (element=w851:string)
        n514 = Concatenate Strings(w850, "\\", w851) -> (w847:string)
        n515 = String To Path(string=w847) -> (path=w846:path)
        n516 = local write "Transfer File"(w846) -> ()
      }
      frame "Previous File" {
        n517 = call "IMAQ Dispose"("All Images? (No)"=TRUE) -> ()  [unwired: 5 in, 1 out]
        n518 = Strip Path(path=w869) -> (stripped path=w866:path, name=w877:string)
        n519 = local write "Transfer Folder"(w866) -> ()
        n520 = List Folder(path=w866) -> (filenames=w870:string[])  [unwired: 3 in, 3 out]
        n521 = Array Size(array=w870) -> (size(s)=w864:i32)
        n522 = Search 1D Array(1D array=w870, element=w877) -> (index of element=w876:i32)  [unwired: 1 in]
        n523 = Decrement(x=w864) -> (x-1=w863:i32)
        n524 = Equal To 0?(x=w876) -> (x = 0?=w875:bool)
        n525 = case shown="True" w875 {
          tunnel: w868 -> [w880 _]
          tunnel: [w879 w881] -> w867
          tunnel: w863 -> [_ w881]
          frame False {
            n526 = Decrement(x=w880) -> (x-1=w879:i32)
          }
          frame True {
          }
        }
        n527 = Path To String(path=w866) -> (string=w865:string)
        n528 = Index Array(array=w870, index=w867) -> (element=w874:string)
        n529 = Concatenate Strings(w865, "\\", w874) -> (w872:string)
        n530 = String To Path(string=w872) -> (path=w871:path)
        n531 = local write "Transfer File"(w871) -> ()
      }
      frame "Discard File" {
        n532 = Strip Path(path=w896) -> (stripped path=w884:path, name=w887:string)
        n533 = property on="Disable Flag" class="Bool (strict)"("Value"=TRUE) -> ()  [unwired: 2 in, 2 out]
        n534 = List Folder(path=w884) -> (filenames=w886:string[])  [unwired: 3 in, 3 out]
        n535 = Search 1D Array(1D array=w886, element=w887) -> (index of element=w893:i32)  [unwired: 1 in]
        n536 = call "IMAQ Dispose"("All Images? (No)"=TRUE) -> ()  [unwired: 5 in, 1 out]
        n537 = String Subset(string=w887, offset (0)=0, length (rest)=1) -> (substring=w890:string)
        n538 = Equal?(x=w890, y="X") -> (x = y?=w888:bool)
        n539 = case shown="False" w888 {
          tunnel: w884 -> [w905 _]
          tunnel: w896 -> [w901 _]
          tunnel: w887 -> [w900 _]
          tunnel: w893 -> [w899 w909]
          tunnel: [w898 w908] -> w885
          frame False {
            n540 = Increment(x=w899) -> (x+1=w898:i32)
            n541 = Path To String(path=w905) -> (string=w904:string)
            n542 = Concatenate Strings(w904, "\\", "X_", w900) -> (w903:string)
            n543 = String To Path(string=w903) -> (path=w902:path)
            n544 = Move(source path=w901, 10:w902) -> ()  [unwired: 3 in, 3 out]
          }
          frame True {
            n545 = Increment(x=w909) -> (x+1=w908:i32)
          }
        }
        n546 = Index Array(array=w886, index=w885) -> (element=w883:string)
        n547 = Build Path(base path=w884, name or relative path=w883) -> (appended path=w882:path)
        n548 = local write "Transfer File"(w882) -> ()
      }
      frame "Save" {
        n549 = Strip Path(path=w913) -> (name=w917:string)  [unwired: 1 out]
        n550 = Search/Split String(string=w917, search string/char (-)="K") -> (match + rest of string=w915:string)  [unwired: 1 in, 2 out]
        n551 = String Subset(string=w915, offset (0)=1) -> (substring=w912:string)  [unwired: 1 in]
        n552 = stacked-sequence {
          seq-local: [w923 _] -> [_ w1405]
          seq-local: [w922 _] -> [_ w1403]
          tunnel: w913 -> [w924 w1406]
          tunnel: w912 -> [w921 _]
          frame #0 {
            # "Saves each Re-calculated parameter in sequence"
            n553 = stacked-sequence {
              tunnel: [_ _ _ _ _ _ _ _ _ _ _ _ _ w1373] -> w922
              tunnel: w924 -> [w944 _ _ _ _ _ _ _ _ _ _ _ _ _]
              frame #0 {
                n554 = call-poly <vilib>:"Read From Spreadsheet File.vi"("file path (dialog if empty)"=w944) -> ("all rows"=w943:string[][])  [unwired: 6 in, 4 out]
                n555 = Array Size(array=w943) -> (size(s)=w948:i32[])
                n556 = Array Subset(array=w943, index (row)=0, index (col)=0, length (col)=3) -> (w952:string[][])  [unwired: 1 in]
                n557 = Index Array(array=w948, index=0) -> (element=w946:i32)
                n558 = Reshape Array(w952, w946) -> (w945:string[])
                n559 = Search 1D Array(1D array=w945, element="Dielectric (nm):") -> (index of element=w955:i32)  [unwired: 1 in]
                n560 = Equal?(x=w955, y=-1) -> (x = y?=w954:bool)
                n561 = case shown="False" w954 {
                  tunnel: w943 -> [w962 w966]
                  tunnel: w955 -> [w960 _]
                  tunnel: [w959 w966] -> w953
                  frame False {
                    n562 = local read "New: Dielectric"() -> (w964:dbl)
                    n563 = Number To Fractional String(number=w964) -> (F-format string=w961:string)  [unwired: 3 in]
                    n564 = Quotient & Remainder(x=w960, y=3) -> (floor(x/y)=w958:i32)  [unwired: 1 out]
                    n565 = Replace Array Subset(array=w962, new element=w961, index (row)=w958, index (col)=1) -> (w959:string[][])
                  }
                  frame True {
                  }
                }
                n566 = local write "Save Array"(w953) -> ()
              }
              frame #1 {
                n567 = local read "Save Array"() -> (w968:string[][])
                n568 = Array Size(array=w968) -> (size(s)=w971:i32[])
                n569 = Array Subset(array=w968, index (row)=0, index (col)=0, length (col)=3) -> (w975:string[][])  [unwired: 1 in]
                n570 = Index Array(array=w971, index=0) -> (element=w969:i32)
                n571 = Reshape Array(w975, w969) -> (w967:string[])
                n572 = Search 1D Array(1D array=w967, element="Comments:") -> (index of element=w978:i32)  [unwired: 1 in]
                n573 = Equal?(x=w978, y=-1) -> (x = y?=w977:bool)
                n574 = case shown="False" w977 {
                  tunnel: w968 -> [w986 w988]
                  tunnel: w978 -> [w983 _]
                  tunnel: [w985 w988] -> w976
                  frame False {
                    n575 = local read "Comments:"() -> (w984:string)
                    n576 = Quotient & Remainder(x=w983, y=3) -> (floor(x/y)=w981:i32)  [unwired: 1 out]
                    n577 = Replace Array Subset(array=w986, new element=w984, index (row)=w981, index (col)=1) -> (w985:string[][])
                  }
                  frame True {
                  }
                }
                n578 = local write "Save Array"(w976) -> ()
              }
              frame #2 {
                n579 = local read "Save Array"() -> (w990:string[][])
                n580 = Array Size(array=w990) -> (size(s)=w993:i32[])
                n581 = Array Subset(array=w990, index (row)=0, index (col)=0, length (col)=3) -> (w997:string[][])  [unwired: 1 in]
                n582 = Index Array(array=w993, index=0) -> (element=w991:i32)
                n583 = Reshape Array(w997, w991) -> (w989:string[])
                n584 = Search 1D Array(1D array=w989, element="Length (um):") -> (index of element=w1000:i32)  [unwired: 1 in]
                n585 = Equal?(x=w1000, y=-1) -> (x = y?=w999:bool)
                n586 = case shown="False" w999 {
                  tunnel: w990 -> [w1009 w1012]
                  tunnel: w1000 -> [w1008 _]
                  tunnel: [w1007 w1012] -> w998
                  frame False {
                    n587 = local read "New: Length"() -> (w1004:dbl)
                    n588 = Quotient & Remainder(x=w1008, y=3) -> (floor(x/y)=w1003:i32)  [unwired: 1 out]
                    n589 = Format Value(format string="%#g", value (0)=w1004) -> (output string=w1005:string)  [unwired: 1 in]
                    n590 = Replace Array Subset(array=w1009, new element=w1005, index (row)=w1003, index (col)=1) -> (w1007:string[][])
                  }
                  frame True {
                  }
                }
                n591 = local write "Save Array"(w998) -> ()
              }
              frame #3 {
                n592 = local read "Save Array"() -> (w1014:string[][])
                n593 = Array Size(array=w1014) -> (size(s)=w1019:i32[])
                n594 = Array Subset(array=w1014, index (row)=0, index (col)=0, length (col)=3) -> (w1015:string[][])  [unwired: 1 in]
                n595 = Index Array(array=w1019, index=0) -> (element=w1021:i32)
                n596 = Reshape Array(w1015, w1021) -> (w1013:string[])
                n597 = Search 1D Array(1D array=w1013, element="Width (um):") -> (index of element=w1024:i32)  [unwired: 1 in]
                n598 = Equal?(x=w1024, y=-1) -> (x = y?=w1023:bool)
                n599 = case shown="False" w1023 {
                  tunnel: w1024 -> [w1033 _]
                  tunnel: w1014 -> [w1032 w1036]
                  tunnel: [w1031 w1036] -> w1022
                  frame False {
                    n600 = local read "New: Width"() -> (w1028:dbl)
                    n601 = Quotient & Remainder(x=w1033, y=3) -> (floor(x/y)=w1027:i32)  [unwired: 1 out]
                    n602 = Format Value(format string="%#g", value (0)=w1028) -> (output string=w1029:string)  [unwired: 1 in]
                    n603 = Replace Array Subset(array=w1032, new element=w1029, index (row)=w1027, index (col)=1) -> (w1031:string[][])
                  }
                  frame True {
                  }
                }
                n604 = local write "Save Array"(w1022) -> ()
              }
              frame #4 {
                w1046 = "Sample Temp (K):"
                n605 = local read "Save Array"() -> (w1038:string[][])
                n606 = Array Size(array=w1038) -> (size(s)=w1043:i32[])
                n607 = Array Subset(array=w1038, index (row)=0, index (col)=0, length (col)=3) -> (w1039:string[][])  [unwired: 1 in]
                n608 = Index Array(array=w1043, index=0) -> (element=w1045:i32)
                n609 = Reshape Array(w1039, w1045) -> (w1037:string[])
                n610 = Search 1D Array(1D array=w1037, element=w1046) -> (index of element=w1049:i32)  [unwired: 1 in]
                n611 = Equal?(x=w1049, y=-1) -> (x = y?=w1048:bool)
                n612 = case shown="False" w1048 {
                  tunnel: w1038 -> [w1057 w1070]
                  tunnel: w1049 -> [w1056 _]
                  tunnel: [w1055 w1069] -> w1047
                  tunnel: w1037 -> [_ w1072]
                  tunnel: w1046 -> [_ w1061]
                  frame False {
                    n613 = local read "New: Temp"() -> (w1053:dbl)
                    n614 = Quotient & Remainder(x=w1056, y=3) -> (floor(x/y)=w1051:i32)  [unwired: 1 out]
                    n615 = Format Value(format string="%#g", value (0)=w1053) -> (output string=w1052:string)  [unwired: 1 in]
                    n616 = Replace Array Subset(array=w1057, new element=w1052, index (row)=w1051, index (col)=1) -> (w1055:string[][])
                  }
                  frame True {
                    n617 = local read "New: Temp"() -> (w1063:dbl)
                    n618 = Search 1D Array(1D array=w1072, element="Width (um):") -> (index of element=w1067:i32)  [unwired: 1 in]
                    n619 = Quotient & Remainder(x=w1067, y=3) -> (floor(x/y)=w1060:i32)  [unwired: 1 out]
                    n620 = Increment(x=w1060) -> (x+1=w1066:i32)
                    n621 = Format Value(format string="%#g", value (0)=w1063) -> (output string=w1062:string)  [unwired: 1 in]
                    n622 = Build Array(w1061, w1062) -> (w1065:string[])
                    n623 = Insert Into Array(array=w1070, index (row)=w1066, new element=w1065) -> (w1069:string[][])  [unwired: 1 in]
                  }
                }
                n624 = local write "Save Array"(w1047) -> ()
              }
              frame #5 {
                w1082 = "Mobility-Sat (cm^2/Vs):"
                n625 = local read "Save Array"() -> (w1074:string[][])
                n626 = Array Size(array=w1074) -> (size(s)=w1079:i32[])
                n627 = Array Subset(array=w1074, index (row)=0, index (col)=0, length (col)=3) -> (w1075:string[][])  [unwired: 1 in]
                n628 = Index Array(array=w1079, index=0) -> (element=w1081:i32)
                n629 = Reshape Array(w1075, w1081) -> (w1073:string[])
                n630 = Search 1D Array(1D array=w1073, element=w1082) -> (index of element=w1085:i32)  [unwired: 1 in]
                n631 = Equal?(x=w1085, y=-1) -> (x = y?=w1084:bool)
                n632 = case shown="False" w1084 {
                  tunnel: w1074 -> [w1094 w1104]
                  tunnel: w1085 -> [w1093 _]
                  tunnel: [w1092 w1103] -> w1083
                  tunnel: w1073 -> [_ w1101]
                  tunnel: w1082 -> [_ w1100]
                  frame False {
                    n633 = local read "Re-Calculated Values Cluster"() -> (w1089:T10)
                    n634 = Unbundle By Name(w1089) -> ("Mobility-Sat"=w1088:dbl)
                    n635 = Quotient & Remainder(x=w1093, y=3) -> (floor(x/y)=w1087:i32)  [unwired: 1 out]
                    n636 = Format Value(format string="%#g", value (0)=w1088) -> (output string=w1090:string)  [unwired: 1 in]
                    n637 = Replace Array Subset(array=w1094, new element=w1090, index (row)=w1087, index (col)=1) -> (w1092:string[][])
                  }
                  frame True {
                    n638 = local read "Re-Calculated Values Cluster"() -> (w1099:T10)
                    n639 = Unbundle By Name(w1099) -> ("Mobility-Sat"=w1098:dbl)
                    n640 = Search 1D Array(1D array=w1101, element="Mobility (cm^2/Vs):") -> (index of element=w1107:i32)  [unwired: 1 in]
                    n641 = Quotient & Remainder(x=w1107, y=3) -> (floor(x/y)=w1097:i32)  [unwired: 1 out]
                    n642 = Format Value(format string="%#g", value (0)=w1098) -> (output string=w1102:string)  [unwired: 1 in]
                    n643 = Build Array(w1100, w1102) -> (w1106:string[])
                    n644 = Replace Array Subset(array=w1104, new element=w1106, index (row)=w1097) -> (w1103:string[][])  [unwired: 1 in]
                  }
                }
                n645 = local write "Save Array"(w1083) -> ()
              }
              frame #6 {
                w1119 = "Mobility-Lin (cm^2/Vs):"
                n646 = local read "Save Array"() -> (w1110:string[][])
                n647 = Array Size(array=w1110) -> (size(s)=w1116:i32[])
                n648 = Array Subset(array=w1110, index (row)=0, index (col)=0, length (col)=3) -> (w1112:string[][])  [unwired: 1 in]
                n649 = Index Array(array=w1116, index=0) -> (element=w1118:i32)
                n650 = Reshape Array(w1112, w1118) -> (w1111:string[])
                n651 = Search 1D Array(1D array=w1111, element=w1119) -> (index of element=w1122:i32)  [unwired: 1 in]
                n652 = Equal?(x=w1122, y=-1) -> (x = y?=w1121:bool)
                n653 = case shown="True" w1121 {
                  tunnel: w1110 -> [w1131 w1140]
                  tunnel: w1122 -> [w1130 _]
                  tunnel: [w1129 w1139] -> w1120
                  tunnel: w1111 -> [_ w1138]
                  tunnel: w1119 -> [_ w1137]
                  frame False {
                    n654 = local read "Re-Calculated Values Cluster"() -> (w1126:T10)
                    n655 = Unbundle By Name(w1126) -> ("Moblitity-Lin"=w1125:dbl)
                    n656 = Quotient & Remainder(x=w1130, y=3) -> (floor(x/y)=w1124:i32)  [unwired: 1 out]
                    n657 = Format Value(format string="%#g", value (0)=w1125) -> (output string=w1127:string)  [unwired: 1 in]
                    n658 = Replace Array Subset(array=w1131, new element=w1127, index (row)=w1124, index (col)=1) -> (w1129:string[][])
                  }
                  frame True {
                    n659 = local read "Re-Calculated Values Cluster"() -> (w1136:T10)
                    n660 = Unbundle By Name(w1136) -> ("Moblitity-Lin"=w1135:dbl)
                    n661 = Search 1D Array(1D array=w1138, element="Mobility-Sat (cm^2/Vs):") -> (index of element=w1144:i32)  [unwired: 1 in]
                    n662 = Quotient & Remainder(x=w1144, y=3) -> (floor(x/y)=w1134:i32)  [unwired: 1 out]
                    n663 = Format Value(format string="%#g", value (0)=w1135) -> (output string=w1147:string)  [unwired: 1 in]
                    n664 = Build Array(w1137, w1147) -> (w1142:string[])
                    n665 = Increment(x=w1134) -> (x+1=w1143:i32)
                    n666 = Insert Into Array(array=w1140, index (row)=w1143, new element=w1142) -> (w1139:string[][])  [unwired: 1 in]
                  }
                }
                n667 = local write "Save Array"(w1120) -> ()
              }
              frame #7 {
                w1157 = "On/Off I-Sat:"
                n668 = local read "Save Array"() -> (w1148:string[][])
                n669 = Array Size(array=w1148) -> (size(s)=w1154:i32[])
                n670 = Array Subset(array=w1148, index (row)=0, index (col)=0, length (col)=3) -> (w1150:string[][])  [unwired: 1 in]
                n671 = Index Array(array=w1154, index=0) -> (element=w1156:i32)
                n672 = Reshape Array(w1150, w1156) -> (w1149:string[])
                n673 = Search 1D Array(1D array=w1149, element=w1157) -> (index of element=w1160:i32)  [unwired: 1 in]
                n674 = Equal?(x=w1160, y=-1) -> (x = y?=w1159:bool)
                n675 = case shown="True" w1159 {
                  tunnel: w1148 -> [w1169 w1178]
                  tunnel: w1160 -> [w1168 _]
                  tunnel: [w1167 w1179] -> w1158
                  tunnel: w1149 -> [_ w1176]
                  tunnel: w1157 -> [_ w1175]
                  frame False {
                    n676 = local read "Calculated Values Cluster"() -> (w1164:T10)
                    n677 = Quotient & Remainder(x=w1168, y=3) -> (floor(x/y)=w1162:i32)  [unwired: 1 out]
                    n678 = Unbundle By Name(w1164) -> ("On/Off"=w1163:dbl)
                    n679 = Format Value(format string="%#g", value (0)=w1163) -> (output string=w1165:string)  [unwired: 1 in]
                    n680 = Replace Array Subset(array=w1169, new element=w1165, index (row)=w1162, index (col)=1) -> (w1167:string[][])
                  }
                  frame True {
                    n681 = local read "Calculated Values Cluster"() -> (w1174:T10)
                    n682 = Unbundle By Name(w1174) -> ("On/Off"=w1173:dbl)
                    n683 = Search 1D Array(1D array=w1176, element="On/Off Current:") -> (index of element=w1182:i32)  [unwired: 1 in]
                    n684 = Quotient & Remainder(x=w1182, y=3) -> (floor(x/y)=w1172:i32)  [unwired: 1 out]
                    n685 = Format Value(format string="%#g", value (0)=w1173) -> (output string=w1177:string)  [unwired: 1 in]
                    n686 = Build Array(w1175, w1177) -> (w1181:string[])
                    n687 = Replace Array Subset(array=w1178, new element=w1181, index (row)=w1172) -> (w1179:string[][])  [unwired: 1 in]
                  }
                }
                n688 = local write "Save Array"(w1158) -> ()
              }
              frame #8 {
                w1194 = "Off I-Sat (A):"
                n689 = local read "Save Array"() -> (w1185:string[][])
                n690 = Array Size(array=w1185) -> (size(s)=w1191:i32[])
                n691 = Array Subset(array=w1185, index (row)=0, index (col)=0, length (col)=3) -> (w1187:string[][])  [unwired: 1 in]
                n692 = Index Array(array=w1191, index=0) -> (element=w1193:i32)
                n693 = Reshape Array(w1187, w1193) -> (w1186:string[])
                n694 = Search 1D Array(1D array=w1186, element=w1194) -> (index of element=w1197:i32)  [unwired: 1 in]
                n695 = Equal?(x=w1197, y=-1) -> (x = y?=w1196:bool)
                n696 = case shown="True" w1196 {
                  tunnel: w1185 -> [w1206 w1215]
                  tunnel: w1197 -> [w1205 _]
                  tunnel: [w1204 w1214] -> w1195
                  tunnel: w1186 -> [_ w1213]
                  tunnel: w1194 -> [_ w1212]
                  frame False {
                    # "New Data File"
                    n697 = local read "Calculated Values Cluster"() -> (w1201:T10)
                    n698 = Unbundle By Name(w1201) -> ("Off Current"=w1200:dbl)
                    n699 = Quotient & Remainder(x=w1205, y=3) -> (floor(x/y)=w1199:i32)  [unwired: 1 out]
                    n700 = Format Value(format string="%#g", value (0)=w1200) -> (output string=w1202:string)  [unwired: 1 in]
                    n701 = Replace Array Subset(array=w1206, new element=w1202, index (row)=w1199, index (col)=1) -> (w1204:string[][])
                  }
                  frame True {
                    # "Old Data File"
                    n702 = local read "Calculated Values Cluster"() -> (w1211:T10)
                    n703 = Unbundle By Name(w1211) -> ("Off Current"=w1210:dbl)
                    n704 = Search 1D Array(1D array=w1213, element="On/Off I-Sat:") -> (index of element=w1219:i32)  [unwired: 1 in]
                    n705 = Quotient & Remainder(x=w1219, y=3) -> (floor(x/y)=w1209:i32)  [unwired: 1 out]
                    n706 = Format Value(format string="%#g", value (0)=w1210) -> (output string=w1222:string)  [unwired: 1 in]
                    n707 = Build Array(w1212, w1222) -> (w1217:string[])
                    n708 = Increment(x=w1209) -> (x+1=w1218:i32)
                    n709 = Insert Into Array(array=w1215, index (row)=w1218, new element=w1217) -> (w1214:string[][])  [unwired: 1 in]
                  }
                }
                n710 = local write "Save Array"(w1195) -> ()
              }
              frame #9 {
                w1224 = "Vt-Sat (V):"
                n711 = local read "Save Array"() -> (w1225:string[][])
                n712 = Array Size(array=w1225) -> (size(s)=w1230:i32[])
                n713 = Array Subset(array=w1225, index (row)=0, index (col)=0, length (col)=3) -> (w1226:string[][])  [unwired: 1 in]
                n714 = Index Array(array=w1230, index=0) -> (element=w1232:i32)
                n715 = Reshape Array(w1226, w1232) -> (w1223:string[])
                n716 = Search 1D Array(1D array=w1223, element=w1224) -> (index of element=w1235:i32)  [unwired: 1 in]
                n717 = Equal?(x=w1235, y=-1) -> (x = y?=w1234:bool)
                n718 = case shown="True" w1234 {
                  tunnel: w1225 -> [w1243 w1255]
                  tunnel: w1235 -> [w1241 _]
                  tunnel: [w1240 w1254] -> w1233
                  tunnel: w1224 -> [_ w1253]
                  tunnel: w1223 -> [_ w1252]
                  frame False {
                    n719 = local read "Re-Calculated Values Cluster"() -> (w1239:T10)
                    n720 = Unbundle By Name(w1239) -> ("Vt-Sat"=w1238:dbl)
                    n721 = Quotient & Remainder(x=w1241, y=3) -> (floor(x/y)=w1237:i32)  [unwired: 1 out]
                    n722 = Number To Fractional String(number=w1238) -> (F-format string=w1242:string)  [unwired: 3 in]
                    n723 = Replace Array Subset(array=w1243, new element=w1242, index (row)=w1237, index (col)=1) -> (w1240:string[][])
                  }
                  frame True {
                    n724 = local read "Re-Calculated Values Cluster"() -> (w1251:T10)
                    n725 = Unbundle By Name(w1251) -> ("Vt-Sat"=w1250:dbl)
                    n726 = Search 1D Array(1D array=w1252, element="Off I-Sat (A):") -> (index of element=w1248:i32)  [unwired: 1 in]
                    n727 = Add(x=w1248, y=3) -> (x+y=w1246:i32)
                    n728 = Quotient & Remainder(x=w1246, y=3) -> (floor(x/y)=w1249:i32)  [unwired: 1 out]
                    n729 = Format Value(format string="%#g", value (0)=w1250) -> (output string=w1260:string)  [unwired: 1 in]
                    n730 = Build Array(w1253, w1260) -> (w1257:string[])
                    n731 = Replace Array Subset(array=w1255, new element=w1257, index (row)=w1249) -> (w1254:string[][])  [unwired: 1 in]
                  }
                }
                n732 = local write "Save Array"(w1233) -> ()
              }
              frame #10 {
                n733 = disable-structure shown="Enabled" {
                  frame Disabled {
                    n734 = local read "Save Array"() -> (w1261:string[][])
                    n735 = Array Size(array=w1261) -> (size(s)=w1267:i32[])
                    n736 = Array Subset(array=w1261, index (row)=0, index (col)=0, length (col)=3) -> (w1263:string[][])  [unwired: 1 in]
                    n737 = Index Array(array=w1267, index=0) -> (element=w1269:i32)
                    n738 = Reshape Array(w1263, w1269) -> (w1262:string[])
                    n739 = Search 1D Array(1D array=w1262, element="VT-Lin (V):") -> (index of element=w1272:i32)  [unwired: 1 in]
                    n740 = Equal?(x=w1272, y=-1) -> (x = y?=w1271:bool)
                    n741 = case shown="True" w1271 {
                      tunnel: w1261 -> [w1280 w1283]
                      tunnel: w1272 -> [w1279 _]
                      tunnel: [w1278 w1283] -> w1270
                      frame False {
                        n742 = Quotient & Remainder(x=w1279, y=3) -> (floor(x/y)=w1275:i32)  [unwired: 1 out]
                        n743 = Format Value(format string="%#g") -> (output string=w1276:string)  [unwired: 2 in]
                        n744 = Replace Array Subset(array=w1280, new element=w1276, index (row)=w1275, index (col)=1) -> (w1278:string[][])
                      }
                      frame True {
                      }
                    }
                    n745 = local write "Save Array"(w1270) -> ()
                  }
                  frame Enabled {
                  }
                }
              }
              frame #11 {
                w1284 = "STS-Sat (V/decade):"
                n746 = local read "Save Array"() -> (w1286:string[][])
                n747 = Array Size(array=w1286) -> (size(s)=w1291:i32[])
                n748 = Array Subset(array=w1286, index (row)=0, index (col)=0, length (col)=3) -> (w1287:string[][])  [unwired: 1 in]
                n749 = Index Array(array=w1291, index=0) -> (element=w1293:i32)
                n750 = Reshape Array(w1287, w1293) -> (w1285:string[])
                n751 = Search 1D Array(1D array=w1285, element=w1284) -> (index of element=w1296:i32)  [unwired: 1 in]
                n752 = Equal?(x=w1296, y=-1) -> (x = y?=w1295:bool)
                n753 = case shown="True" w1295 {
                  tunnel: w1286 -> [w1305 w1316]
                  tunnel: w1296 -> [w1304 _]
                  tunnel: [w1303 w1317] -> w1294
                  tunnel: w1285 -> [_ w1315]
                  tunnel: w1284 -> [_ w1314]
                  frame False {
                    # "Current Data File"
                    n754 = local read "Re-Calculated Values Cluster"() -> (w1299:T10)
                    n755 = Unbundle By Name(w1299) -> ("STS"=w1300:dbl)
                    n756 = Quotient & Remainder(x=w1304, y=3) -> (floor(x/y)=w1298:i32)  [unwired: 1 out]
                    n757 = Format Value(format string="%#g", value (0)=w1300) -> (output string=w1301:string)  [unwired: 1 in]
                    n758 = Replace Array Subset(array=w1305, new element=w1301, index (row)=w1298, index (col)=1) -> (w1303:string[][])
                  }
                  frame True {
                    # "Old Data File"
                    n759 = local read "Re-Calculated Values Cluster"() -> (w1312:T10)
                    n760 = Unbundle By Name(w1312) -> ("STS"=w1313:dbl)
                    n761 = Search 1D Array(1D array=w1315, element="Vt-Sat (V):") -> (index of element=w1309:i32)  [unwired: 1 in]
                    n762 = Add(x=w1309, y=3) -> (x+y=w1308:i32)
                    n763 = Quotient & Remainder(x=w1308, y=3) -> (floor(x/y)=w1311:i32)  [unwired: 1 out]
                    n764 = Format Value(format string="%#g", value (0)=w1313) -> (output string=w1322:string)  [unwired: 1 in]
                    n765 = Build Array(w1314, w1322) -> (w1319:string[])
                    n766 = Replace Array Subset(array=w1316, new element=w1319, index (row)=w1311) -> (w1317:string[][])  [unwired: 1 in]
                  }
                }
                n767 = local write "Save Array"(w1294) -> ()
              }
              frame #12 {
                w1323 = "Trap Density-VT (Traps/Vcm^2):"
                n768 = local read "Save Array"() -> (w1325:string[][])
                n769 = Array Size(array=w1325) -> (size(s)=w1330:i32[])
                n770 = Array Subset(array=w1325, index (row)=0, index (col)=0, length (col)=3) -> (w1326:string[][])  [unwired: 1 in]
                n771 = Index Array(array=w1330, index=0) -> (element=w1332:i32)
                n772 = Reshape Array(w1326, w1332) -> (w1324:string[])
                n773 = Search 1D Array(1D array=w1324, element=w1323) -> (index of element=w1335:i32)  [unwired: 1 in]
                n774 = Equal?(x=w1335, y=-1) -> (x = y?=w1334:bool)
                n775 = case shown="True" w1334 {
                  tunnel: w1325 -> [w1344 w1355]
                  tunnel: w1335 -> [w1342 _]
                  tunnel: [w1341 w1356] -> w1333
                  tunnel: w1324 -> [_ w1354]
                  tunnel: w1323 -> [_ w1353]
                  frame False {
                    n776 = local read "Re-Calculated Values Cluster"() -> (w1339:T10)
                    n777 = Unbundle By Name(w1339) -> ("Trap Density-VT"=w1338:dbl)
                    n778 = Quotient & Remainder(x=w1342, y=3) -> (floor(x/y)=w1337:i32)  [unwired: 1 out]
                    n779 = Format Value(format string="%#g", value (0)=w1338) -> (output string=w1343:string)  [unwired: 1 in]
                    n780 = Replace Array Subset(array=w1344, new element=w1343, index (row)=w1337, index (col)=1) -> (w1341:string[][])
                  }
                  frame True {
                    n781 = local read "Re-Calculated Values Cluster"() -> (w1352:T10)
                    n782 = Unbundle By Name(w1352) -> ("Trap Density-VT"=w1351:dbl)
                    n783 = Search 1D Array(1D array=w1354, element="STS-Sat (V/decade):") -> (index of element=w1348:i32)  [unwired: 1 in]
                    n784 = Add(x=w1348, y=3) -> (x+y=w1347:i32)
                    n785 = Quotient & Remainder(x=w1347, y=3) -> (floor(x/y)=w1350:i32)  [unwired: 1 out]
                    n786 = Format Value(format string="%#g", value (0)=w1351) -> (output string=w1357:string)  [unwired: 1 in]
                    n787 = Build Array(w1353, w1357) -> (w1361:string[])
                    n788 = Increment(x=w1350) -> (x+1=w1360:i32)
                    n789 = Insert Into Array(array=w1355, index (row)=w1360, new element=w1361) -> (w1356:string[][])  [unwired: 1 in]
                  }
                }
                n790 = local write "Save Array"(w1333) -> ()
              }
              frame #13 {
                w1363 = "Trap Density-STS (Traps/Vcm^2):"
                n791 = local read "Save Array"() -> (w1365:string[][])
                n792 = Array Size(array=w1365) -> (size(s)=w1370:i32[])
                n793 = Array Subset(array=w1365, index (row)=0, index (col)=0, length (col)=3) -> (w1366:string[][])  [unwired: 1 in]
                n794 = Index Array(array=w1370, index=0) -> (element=w1372:i32)
                n795 = Reshape Array(w1366, w1372) -> (w1364:string[])
                n796 = Search 1D Array(1D array=w1364, element=w1363) -> (index of element=w1375:i32)  [unwired: 1 in]
                n797 = Equal?(x=w1375, y=-1) -> (x = y?=w1374:bool)
                n798 = case shown="True" w1374 {
                  tunnel: w1365 -> [w1384 w1395]
                  tunnel: w1375 -> [w1383 _]
                  tunnel: [w1382 w1396] -> w1373
                  tunnel: w1364 -> [_ w1394]
                  tunnel: w1363 -> [_ w1393]
                  frame False {
                    n799 = local read "Re-Calculated Values Cluster"() -> (w1379:T10)
                    n800 = Unbundle By Name(w1379) -> ("Trap Density-STS"=w1378:dbl)
                    n801 = Quotient & Remainder(x=w1383, y=3) -> (floor(x/y)=w1377:i32)  [unwired: 1 out]
                    n802 = Format Value(format string="%#g", value (0)=w1378) -> (output string=w1380:string)  [unwired: 1 in]
                    n803 = Replace Array Subset(array=w1384, new element=w1380, index (row)=w1377, index (col)=1) -> (w1382:string[][])
                  }
                  frame True {
                    n804 = local read "Re-Calculated Values Cluster"() -> (w1392:T10)
                    n805 = Unbundle By Name(w1392) -> ("Trap Density-STS"=w1391:dbl)
                    n806 = Search 1D Array(1D array=w1394, element="Trap Density-VT (Traps/Vcm^2):") -> (index of element=w1388:i32)  [unwired: 1 in]
                    n807 = Add(x=w1388, y=3) -> (x+y=w1387:i32)
                    n808 = Quotient & Remainder(x=w1387, y=3) -> (floor(x/y)=w1390:i32)  [unwired: 1 out]
                    n809 = Format Value(format string="%#g", value (0)=w1391) -> (output string=w1402:string)  [unwired: 1 in]
                    n810 = Build Array(w1393, w1402) -> (w1398:string[])
                    n811 = Increment(x=w1390) -> (x+1=w1399:i32)
                    n812 = Insert Into Array(array=w1395, index (row)=w1399, new element=w1398) -> (w1396:string[][])  [unwired: 1 in]
                  }
                }
                n813 = local write "Save Array"(w1373) -> ()
              }
            }
            n814 = local read "New: Temp"() -> (w925:dbl)
            n815 = local read "New: Width"() -> (w926:dbl)
            n816 = local read "New: Length"() -> (w928:dbl)
            n817 = local read "Index"() -> (w927:string)
            n818 = To Long Integer(number=w925) -> (32bit integer=w942:i32)
            n819 = Number To Decimal String(number=w942) -> (decimal integer string=w937:string)  [unwired: 1 in]
            n820 = To Long Integer(number=w926) -> (32bit integer=w941:i32)
            n821 = To Long Integer(number=w928) -> (32bit integer=w940:i32)
            n822 = Strip Path(path=w924) -> (stripped path=w929:path)  [unwired: 1 out]
            n823 = Number To Decimal String(number=w940) -> (decimal integer string=w935:string)  [unwired: 1 in]
            n824 = Number To Decimal String(number=w941) -> (decimal integer string=w934:string)  [unwired: 1 in]
            n825 = Concatenate Strings("_", w937, "K") -> (w939:string)
            n826 = call "Build Text"("Temp"=w939, "Index"=w927, "Length"=w935, "Width"=w934) -> ("Result"=w933:string)  [unwired: 10 in, 1 out]
            n827 = Path To String(path=w929) -> (string=w931:string)
            n828 = Concatenate Strings(w931, "\\", w933, w921) -> (w932:string)
            n829 = String To Path(string=w932) -> (path=w923:path)
          }
          frame #1 {
            n830 = flat-sequence {
              tunnel: w1406 -> [w1408]
              tunnel: w1405 -> [w1407]
              tunnel: [w1407] -> w1404
              tunnel: w1404 -> [w1414]
              tunnel: w1403 -> [w1413]
              frame #0 {
                n831 = Equal?(x=w1408, y=w1407) -> (x = y?=w1409:bool)
                n832 = case shown="False" w1409 {
                  tunnel: w1408 -> [w1412 _]
                  tunnel: w1407 -> [w1411 _]
                  frame False {
                    n833 = Move(source path=w1412, 9:TRUE, 10:w1411) -> ()  [unwired: 2 in, 3 out]
                  }
                  frame True {
                  }
                }
              }
              frame #1 {
                n834 = local write "Transfer File"(w1414) -> ()
                n835 = call-poly <vilib>:"Write To Spreadsheet File.vi"("2D data"=w1413, "file path (dialog if empty)"=w1414) -> ()  [unwired: 6 in, 1 out]
              }
            }
          }
        }
        n836 = local read "Save Next?"() -> (w918:bool)
        n837 = Select(t=MegaAwesome_States."Next File", s=w918, f=MegaAwesome_States."No Event") -> (s? t:f=w919:T2)
      }
      frame "Exit" {
        n838 = disable-structure shown="Disabled" {
          disable-tunnel: [w1418 _] -> _
          disable-tunnel: [w1417 _] -> _
          frame Disabled {
            n839 = flat-sequence {
              tunnel: [w1427] -> w1418
              tunnel: [w1427] -> w1417
              frame #0 {
                w1426 = FALSE
                n840 = property on="Next File" class="Bool (strict)"("Value"=w1426) -> (error out=w1421:errorcluster)  [unwired: 2 in, 1 out]
                n841 = property on="Previous File" class="Bool (strict)"(error in=w1421, "Value"=w1426) -> (error out=w1422:errorcluster)  [unwired: 1 in, 1 out]
                n842 = Request Deallocation(TRUE) -> ()
                n843 = property on="Save" class="Bool (strict)"(error in=w1422, "Value"=w1426) -> (error out=w1423:errorcluster)  [unwired: 1 in, 1 out]
                n844 = property on="Export" class="Bool (strict)"("Value"=w1426) -> ()  [unwired: 2 in, 2 out]
                n845 = property on="Save Next" class="Bool (strict)"(error in=w1423, "Value"=w1426) -> (error out=w1424:errorcluster)  [unwired: 1 in, 1 out]
                n846 = property on="Discard" class="Bool (strict)"(error in=w1424, "Value"=w1426) -> (error out=w1425:errorcluster)  [unwired: 1 in, 1 out]
                n847 = property on="Save Lines" class="Bool (strict)"(error in=w1425, "Value"=w1426) -> ()  [unwired: 1 in, 2 out]
                n848 = property on="Close" class="Bool (strict)"("Value"=w1426) -> ()  [unwired: 2 in, 2 out]
                n849 = property on="Disable Flag" class="Bool (strict)"("Value"=w1426) -> ()  [unwired: 2 in, 2 out]
                n850 = call "IMAQ Dispose"("All Images? (No)"=TRUE) -> ()  [unwired: 5 in, 1 out]
              }
              frame #1 {
                w1427 = MegaAwesome_States."Exit"
              }
            }
          }
          frame Enabled {
          }
        }
        n851 = event shown="[0] Application Instance Close?" {
          selector: _ -> [_]
          dyn-events: _ -> [_]
          timeout: _ -> [_]
          event Application Instance Close? {
            n852 = event-data() -> ()  [unwired: 1 in, 4 out]
            n853 = event-data("Discard?"=TRUE) -> ()  [unwired: 2 in, 1 out]
          }
        }
      }
      frame "Save Lines" {
        n854 = Build Path(base path=w1430, name or relative path="ROI") -> (appended path=w1433:path)
        n855 = call <vilib>:"Check if File or Folder Exists.vi"("path"=w1433) -> ("file or folder exists?"=w1431:bool, "dup path"=w1434:path)  [unwired: 8 in, 1 out]
        n856 = case shown="False" w1431 {
          tunnel: w1434 -> [w1442 w1443]
          tunnel: [w1441 w1443] -> w1438
          frame False {
            n857 = Create Folder(path (use dialog)=w1442) -> (created path=w1441:path)  [unwired: 2 in, 2 out]
          }
          frame True {
          }
        }
        n858 = local read "Index"() -> (w1429:string)
        n859 = property on="Image Out" class="ImageControl"() -> ("ROI"=w1435:T21)  [unwired: 2 in, 2 out]
        n860 = Build Path(base path=w1438, name or relative path=w1429) -> (appended path=w1437:path)
        n861 = Flatten To String(anything=w1435) -> (data string=w1436:string)  [unwired: 3 in, 2 out]
        n862 = Write to Text File(file (use dialog)=w1437, text=w1436) -> ()  [unwired: 2 in, 3 out]
      }
      frame "Export" {
        n863 = flat-sequence {
          tunnel: ["Independant Variable:"] -> w1445
          tunnel: w1444 -> [w1448]
          tunnel: w1445 -> [w1527]
          frame #0 {
            n864 = stacked-sequence {
              tunnel: "Independant Variable:" -> [w1450 w1456 w1462 w1468 w1474 w1480 w1486 w1492 w1498 w1504 w1511]
              tunnel: w1448 -> [_ _ _ _ _ _ _ _ _ _ w1510]
              frame #0 {
                n865 = Equal?(x=w1450, y="Length (um):") -> (x = y?=w1451:bool)
                n866 = case shown="True" w1451 {
                  frame False {
                  }
                  frame True {
                    n867 = local write "X Axis Display Type"("1") -> ()
                    n868 = local write "Opj X Axis"("2") -> ()
                    n869 = local write "Stats Label"("Length" ("Stats Label")) -> ()
                  }
                }
              }
              frame #1 {
                n870 = Equal?(x=w1456, y="Sample Temp (K):") -> (x = y?=w1457:bool)
                n871 = case shown="True" w1457 {
                  frame False {
                  }
                  frame True {
                    n872 = local write "X Axis Display Type"("1") -> ()
                    n873 = local write "Stats Label"("Temp" ("Stats Label")) -> ()
                    n874 = local write "Opj X Axis"("1") -> ()
                  }
                }
              }
              frame #2 {
                n875 = Equal?(x=w1462, y="Mobility-Sat (cm^2/Vs):") -> (x = y?=w1463:bool)
                n876 = case shown="True" w1463 {
                  frame False {
                  }
                  frame True {
                    n877 = local write "X Axis Display Type"("2") -> ()
                    n878 = local write "Opj X Axis"("2") -> ()
                    n879 = local write "Stats Label"("Mob-Sat" ("Stats Label")) -> ()
                  }
                }
              }
              frame #3 {
                n880 = Equal?(x=w1468, y="Mobility-Lin (cm^2/Vs):") -> (x = y?=w1469:bool)
                n881 = case shown="True" w1469 {
                  frame False {
                  }
                  frame True {
                    n882 = local write "X Axis Display Type"("2") -> ()
                    n883 = local write "Opj X Axis"("2") -> ()
                    n884 = local write "Stats Label"("Mob-Lin" ("Stats Label")) -> ()
                  }
                }
              }
              frame #4 {
                n885 = Equal?(x=w1474, y="On/Off I-Sat:") -> (x = y?=w1475:bool)
                n886 = case shown="True" w1475 {
                  frame False {
                  }
                  frame True {
                    n887 = local write "X Axis Display Type"("2") -> ()
                    n888 = local write "Opj X Axis"("2") -> ()
                    n889 = local write "Stats Label"("On-Off I" ("Stats Label")) -> ()
                  }
                }
              }
              frame #5 {
                n890 = Equal?(x=w1480, y="Off I-Sat (A):") -> (x = y?=w1481:bool)
                n891 = case shown="True" w1481 {
                  frame False {
                  }
                  frame True {
                    n892 = local write "X Axis Display Type"("2") -> ()
                    n893 = local write "Stats Label"("Off-I" ("Stats Label")) -> ()
                    n894 = local write "Opj X Axis"("2") -> ()
                  }
                }
              }
              frame #6 {
                n895 = Equal?(x=w1486, y="Vt-Sat (V):") -> (x = y?=w1487:bool)
                n896 = case shown="True" w1487 {
                  frame False {
                  }
                  frame True {
                    n897 = local write "X Axis Display Type"("1") -> ()
                    n898 = local write "Opj X Axis"("1") -> ()
                    n899 = local write "Stats Label"("VT" ("Stats Label")) -> ()
                  }
                }
              }
              frame #7 {
                n900 = Equal?(x=w1492, y="STS-Sat (V/decade):") -> (x = y?=w1493:bool)
                n901 = case shown="True" w1493 {
                  frame False {
                  }
                  frame True {
                    n902 = local write "Opj X Axis"("1") -> ()
                    n903 = local write "X Axis Display Type"("1") -> ()
                    n904 = local write "Stats Label"("STS" ("Stats Label")) -> ()
                  }
                }
              }
              frame #8 {
                n905 = Equal?(x=w1498, y="Trap Density-VT (Traps/Vcm^2):") -> (x = y?=w1499:bool)
                n906 = case shown="True" w1499 {
                  frame False {
                  }
                  frame True {
                    n907 = local write "X Axis Display Type"("2") -> ()
                    n908 = local write "Stats Label"("N-VT" ("Stats Label")) -> ()
                    n909 = local write "Opj X Axis"("2") -> ()
                  }
                }
              }
              frame #9 {
                n910 = Equal?(x=w1504, y="Trap Density-STS (Traps/Vcm^2):") -> (x = y?=w1505:bool)
                n911 = case shown="True" w1505 {
                  frame False {
                  }
                  frame True {
                    n912 = local write "X Axis Display Type"("2") -> ()
                    n913 = local write "Stats Label"("N-STS" ("Stats Label")) -> ()
                    n914 = local write "Opj X Axis"("2") -> ()
                  }
                }
              }
              frame #10 {
                n915 = Equal?(x=w1511, y="Time Stamp:") -> (x = y?=w1512:bool)
                n916 = case shown="True" w1512 {
                  tunnel: w1510 -> [_ w1517]
                  frame False {
                  }
                  frame True {
                    n917 = Strip Path(path=w1517) -> (stripped path=w1516:path)  [unwired: 1 out]
                    n918 = Build Path(base path=w1516, name or relative path="Origin Template_Time.opj") -> (appended path=w1514:path)
                    n919 = local write "X Axis Display Type"("1") -> ()
                    n920 = local write "Origin Project File"(w1514) -> ()
                    n921 = local write "Stats Label"("Time Stamp" ("Stats Label")) -> ()
                    n922 = local write "Opj X Axis"("1") -> ()
                  }
                }
              }
            }
          }
          frame #1 {
            n923 = local read "Stats Label"() -> (w1524:string)
            n924 = local read "Transfer Folder"() -> (w1531:path)
            n925 = Concatenate Strings("Stats", "_" ("string"), w1524) -> (w1522:string)
            n926 = Build Path(base path=w1531, name or relative path=w1522) -> (appended path=w1532:path)
            n927 = local read "Origin Project File"() -> (w1521:path)
            n928 = call <vilib>:"Check if File or Folder Exists.vi"("path"=w1532) -> ("file or folder exists?"=w1546:bool, "dup path"=w1545:path)  [unwired: 8 in, 1 out]
            n929 = call "OA_ConnectToOrigin.vi"() -> ("error out"=w1543:errorcluster, "Origin.IOApplication"=w1544:refnum<k7>)  [unwired: 8 in]
            n930 = case shown="False" w1546 {
              tunnel: w1545 -> [w1718 w1719]
              tunnel: [w1717 w1719] -> w1530
              frame False {
                n931 = Create Folder(path (use dialog)=w1718) -> (created path=w1717:path)  [unwired: 2 in, 2 out]
              }
              frame True {
              }
            }
            n932 = call "File Dialog"("start path"=w1532) -> ("selected path"=w1534:path)  [unwired: 11 in, 3 out]
            n933 = call "OA_Load.vi"("error in (no error)"=w1543, "Path"=w1521, "Origin.IOApplication"=w1544) -> ("error out"=w1541:errorcluster, "Origin.IOApplication"=w1542:refnum<k7>)  [unwired: 1 out]
            n934 = call "OAExecute.vi"("script"="document -m 3;", "Error IO"=w1541, "Origin.IOApplication"=w1542) -> ("Error IO Out"=w1539:errorcluster, "Origin.IOApplication"=w1540:refnum<k7>)  [unwired: 1 in, 1 out]
            n935 = stacked-sequence {
              tunnel: w1531 -> [w1556 w1586 w1598 w1620 w1640 w1661 w1682 w1705]
              tunnel: w1530 -> [w1557 w1585 w1599 w1619 w1641 w1662 w1683 w1706]
              tunnel: w1540 -> [w1559 w1583 w1601 w1622 w1643 w1664 w1685 w1708]
              tunnel: w1539 -> [w1558 w1584 w1600 w1621 w1642 w1663 w1684 w1707]
              tunnel: [_ _ _ _ _ _ _ w1703] -> w1529
              tunnel: [_ _ _ _ _ _ _ w1704] -> w1528
              tunnel: w1527 -> [w1555 w1576 w1597 w1618 w1639 w1660 w1681 w1702]
              frame #0 {
                n936 = local read "X Axis Display Type"() -> (w1547:string)
                n937 = local read "Opj X Axis"() -> (w1552:string)
                n938 = Concatenate Strings("window -a MOBLGraph;\nlayer.x.type=", w1552, "; layer.x.label.numFormat = ", w1547, "; Y3 = 1; X3 = 1;", "window -a MOBLTable;\nwindow -s TV;") -> (w1550:string)
                n939 = call "Param_Analysis_7_24b_JW.vi"("Independant Variable"=w1555, "error in (no error)"=w1558, "Data Folder"=w1556, "Parameter String"="Mobility-Lin (cm^2/Vs):", "Parameter Name"="Mobility-Lin", "Stats Folder"=w1557) -> ("error out"=w1561:errorcluster, "Output Array"=w1563:string[][], "Variables"=w1554:T31)  [unwired: 2 in, 1 out]
                n940 = call "Origin_Export_2014 05 02_JWa.vi"("Input Conditions"=w1554, "Analysis Array"=w1563, "error in (no error)"=w1561, "Parameter Worksheet Name"="[MOBLTable]Mobilities", "Parameter Folder Script"="pe_cd \"Mobility-Lin\";", "Origin.IOApplication"=w1559) -> ("error out"=w1560:errorcluster, "reference out"=w1562:refnum<k7>)  [unwired: 3 in, 1 out]
                n941 = call "OAExecute.vi"("script"=w1550, "Error IO"=w1560, "Origin.IOApplication"=w1562) -> ()  [unwired: 1 in, 3 out]
              }
              frame #1 {
                n942 = local read "X Axis Display Type"() -> (w1568:string)
                n943 = local read "Opj X Axis"() -> (w1573:string)
                n944 = Concatenate Strings("window -a MOBSGraph;\nlayer.x.type=", w1573, "; layer.x.label.numFormat = ", w1568, "; Y3 = 1; X3 = 1;", "window -a MOBSTable;\nwindow -s TV;") -> (w1571:string)
                n945 = call "Param_Analysis_7_24b_JW.vi"("Independant Variable"=w1576, "error in (no error)"=w1584, "Data Folder"=w1586, "Parameter String"="Mobility-Sat (cm^2/Vs):", "Parameter Name"="Mobility-Sat", "Stats Folder"=w1585) -> ("error out"=w1579:errorcluster, "Output Array"=w1577:string[][], "Variables"=w1575:T31)  [unwired: 2 in, 1 out]
                n946 = call "Origin_Export_2014 05 02_JWa.vi"("Input Conditions"=w1575, "Analysis Array"=w1577, "error in (no error)"=w1579, "Parameter Worksheet Name"="[MOBSTable]Mobilities", "Parameter Folder Script"="pe_cd \"Mobility-Sat\";", "Origin.IOApplication"=w1583) -> ("error out"=w1578:errorcluster, "reference out"=w1580:refnum<k7>)  [unwired: 3 in, 1 out]
                n947 = call "OAExecute.vi"("script"=w1571, "Error IO"=w1578, "Origin.IOApplication"=w1580) -> ()  [unwired: 1 in, 3 out]
              }
              frame #2 {
                n948 = local read "X Axis Display Type"() -> (w1589:string)
                n949 = local read "Opj X Axis"() -> (w1594:string)
                n950 = Concatenate Strings("window -a NSTSGraph;\nlayer.x.type=", w1594, "; layer.x.label.numFormat = ", w1589, "; Y3 = 1; X3 = 1;", "window -a NSTSTable;\nwindow -s TV;") -> (w1592:string)
                n951 = call "Param_Analysis_7_24b_JW.vi"("Independant Variable"=w1597, "error in (no error)"=w1600, "Data Folder"=w1598, "Parameter String"="Trap Density-STS (Traps/Vcm^2):", "Parameter Name"="Trap Density-STS", "Stats Folder"=w1599) -> ("error out"=w1604:errorcluster, "Output Array"=w1602:string[][], "Variables"=w1596:T31)  [unwired: 2 in, 1 out]
                n952 = call "Origin_Export_2014 05 02_JWa.vi"("Input Conditions"=w1596, "Analysis Array"=w1602, "error in (no error)"=w1604, "Parameter Worksheet Name"="[NSTSTable]Trap Densities", "Parameter Folder Script"="pe_cd \"N-STS\";", "Origin.IOApplication"=w1601) -> ("error out"=w1603:errorcluster, "reference out"=w1605:refnum<k7>)  [unwired: 3 in, 1 out]
                n953 = call "OAExecute.vi"("script"=w1592, "Error IO"=w1603, "Origin.IOApplication"=w1605) -> ()  [unwired: 1 in, 3 out]
              }
              frame #3 {
                n954 = local read "X Axis Display Type"() -> (w1610:string)
                n955 = local read "Opj X Axis"() -> (w1615:string)
                n956 = call "Param_Analysis_7_24b_JW.vi"("Independant Variable"=w1618, "error in (no error)"=w1621, "Data Folder"=w1620, "Parameter String"="Trap Density-VT (Traps/Vcm^2):", "Parameter Name"="Trap Density-Vt", "Stats Folder"=w1619) -> ("error out"=w1625:errorcluster, "Output Array"=w1623:string[][], "Variables"=w1617:T31)  [unwired: 2 in, 1 out]
                n957 = Concatenate Strings("window -a NVtGraph;\nlayer.x.type=", w1615, "; layer.x.label.numFormat = ", w1610, "; Y3 = 1; X3 = 1;", "window -a NVtTable;\nwindow -s TV;") -> (w1613:string)
                n958 = call "Origin_Export_2014 05 02_JWa.vi"("Input Conditions"=w1617, "Analysis Array"=w1623, "error in (no error)"=w1625, "Parameter Worksheet Name"="[NVTTable]Trap Densities", "Parameter Folder Script"="pe_cd \"N-Vt\";", "Origin.IOApplication"=w1622) -> ("error out"=w1624:errorcluster, "reference out"=w1626:refnum<k7>)  [unwired: 3 in, 1 out]
                n959 = call "OAExecute.vi"("script"=w1613, "Error IO"=w1624, "Origin.IOApplication"=w1626) -> ()  [unwired: 1 in, 3 out]
              }
              frame #4 {
                n960 = local read "X Axis Display Type"() -> (w1631:string)
                n961 = local read "Opj X Axis"() -> (w1636:string)
                n962 = Concatenate Strings("window -a OffIGraph;\nlayer.x.type=", w1636, "; layer.x.label.numFormat = ", w1631, "; Y3 = 1; X3 = 1;", "window -a OffITable;\nwindow -s TV;") -> (w1634:string)
                n963 = call "Param_Analysis_7_24b_JW.vi"("Independant Variable"=w1639, "error in (no error)"=w1642, "Data Folder"=w1640, "Parameter String"="Off I-Sat (A):", "Parameter Name"="Off I-Sat", "Stats Folder"=w1641) -> ("error out"=w1646:errorcluster, "Output Array"=w1644:string[][], "Variables"=w1638:T31)  [unwired: 2 in, 1 out]
                n964 = call "Origin_Export_2014 05 02_JWa.vi"("Input Conditions"=w1638, "Analysis Array"=w1644, "error in (no error)"=w1646, "Parameter Worksheet Name"="[OffItable]OffCurrents", "Parameter Folder Script"="pe_cd \"OffI-Sat\";", "Origin.IOApplication"=w1643) -> ("error out"=w1645:errorcluster, "reference out"=w1647:refnum<k7>)  [unwired: 3 in, 1 out]
                n965 = call "OAExecute.vi"("script"=w1634, "Error IO"=w1645, "Origin.IOApplication"=w1647) -> ()  [unwired: 1 in, 3 out]
              }
              frame #5 {
                n966 = local read "X Axis Display Type"() -> (w1652:string)
                n967 = local read "Opj X Axis"() -> (w1657:string)
                n968 = Concatenate Strings("window -a OnOffGraph;\nlayer.x.type=", w1657, "; layer.x.label.numFormat = ", w1652, "; Y3 = 1; X3 = 1;", "window -a OnOffTable;\nwindow -s TV;") -> (w1655:string)
                n969 = call "Param_Analysis_7_24b_JW.vi"("Independant Variable"=w1660, "error in (no error)"=w1663, "Data Folder"=w1661, "Parameter String"="On/Off I-Sat:", "Parameter Name"="OnOff Ratio", "Stats Folder"=w1662) -> ("error out"=w1667:errorcluster, "Output Array"=w1665:string[][], "Variables"=w1659:T31)  [unwired: 2 in, 1 out]
                n970 = call "Origin_Export_2014 05 02_JWa.vi"("Input Conditions"=w1659, "Analysis Array"=w1665, "error in (no error)"=w1667, "Parameter Worksheet Name"="[OnOffTable]On/Off Ratios", "Parameter Folder Script"="pe_cd \"OnOff-Ratio\";", "Origin.IOApplication"=w1664) -> ("error out"=w1666:errorcluster, "reference out"=w1668:refnum<k7>)  [unwired: 3 in, 1 out]
                n971 = call "OAExecute.vi"("script"=w1655, "Error IO"=w1666, "Origin.IOApplication"=w1668) -> ()  [unwired: 1 in, 3 out]
              }
              frame #6 {
                n972 = local read "X Axis Display Type"() -> (w1673:string)
                n973 = local read "Opj X Axis"() -> (w1678:string)
                n974 = call "Param_Analysis_7_24b_JW.vi"("Independant Variable"=w1681, "error in (no error)"=w1684, "Data Folder"=w1682, "Parameter String"="STS-Sat (V/decade):", "Parameter Name"="STS-Sat", "Stats Folder"=w1683) -> ("error out"=w1688:errorcluster, "Output Array"=w1686:string[][], "Variables"=w1680:T31)  [unwired: 2 in, 1 out]
                n975 = Concatenate Strings("window -a SGraph;\nlayer.x.type=", w1678, "; layer.x.label.numFormat = ", w1673, "; Y3 = 1; X3 = 1;", "window -a STable;\nwindow -s TV;") -> (w1676:string)
                n976 = call "Origin_Export_2014 05 02_JWa.vi"("Input Conditions"=w1680, "Analysis Array"=w1686, "error in (no error)"=w1688, "Parameter Worksheet Name"="[STable]Threshold Swing", "Parameter Folder Script"="pe_cd \"STS-Sat\";", "Origin.IOApplication"=w1685) -> ("error out"=w1687:errorcluster, "reference out"=w1689:refnum<k7>)  [unwired: 3 in, 1 out]
                n977 = call "OAExecute.vi"("script"=w1676, "Error IO"=w1687, "Origin.IOApplication"=w1689) -> ()  [unwired: 1 in, 3 out]
              }
              frame #7 {
                n978 = local read "X Axis Display Type"() -> (w1694:string)
                n979 = local read "Opj X Axis"() -> (w1699:string)
                n980 = Concatenate Strings("window -a VtGraph;\nlayer.x.type=", w1699, "; layer.x.label.numFormat = ", w1694, "; Y3 = 1; X3 = 1;", "window -a VtTable;\nwindow -s TV;") -> (w1697:string)
                n981 = call "Param_Analysis_7_24b_JW.vi"("Independant Variable"=w1702, "error in (no error)"=w1707, "Data Folder"=w1705, "Parameter String"="Vt-Sat (V):", "Parameter Name"="Vt-Sat", "Stats Folder"=w1706) -> ("error out"=w1711:errorcluster, "Output Array"=w1709:string[][], "Variables"=w1701:T31)  [unwired: 2 in, 1 out]
                n982 = call "Origin_Export_2014 05 02_JWa.vi"("Input Conditions"=w1701, "Analysis Array"=w1709, "error in (no error)"=w1711, "Parameter Worksheet Name"="[VtTable]Threshold Voltages", "Parameter Folder Script"="pe_cd \"Vt-Sat\";", "Origin.IOApplication"=w1708) -> ("error out"=w1710:errorcluster, "reference out"=w1712:refnum<k7>)  [unwired: 3 in, 1 out]
                n983 = call "OAExecute.vi"("script"=w1697, "Error IO"=w1710, "Origin.IOApplication"=w1712) -> ("Error IO Out"=w1703:errorcluster, "Origin.IOApplication"=w1704:refnum<k7>)  [unwired: 1 in, 1 out]
              }
            }
            n984 = Path To String(path=w1534) -> (string=w1533:string)
            n985 = call "OAExecute.vi"("script"="pe_cd /; ", "Error IO"=w1529, "Origin.IOApplication"=w1528) -> ("Error IO Out"=w1535:errorcluster, "Origin.IOApplication"=w1536:refnum<k7>)  [unwired: 1 in, 1 out]
            n986 = call "OASaveProject.vi"("path"=w1533, "Error IO"=w1535, "Origin.IOApplication"=w1536) -> ("Origin.IOApplication"=w1526:refnum<k7>)  [unwired: 2 out]
            n987 = call "OAEndSession.vi"("Origin.IOApplication"=w1526) -> ()  [unwired: 1 in, 3 out]
          }
        }
      }
    }
    "Current State" <- w17
    "Folder Index" <- w16
    n988 = Wait (ms)(milliseconds to wait=u32 0) -> ()  [unwired: 1 out]
    n989 = Equal?(x=w17, y=MegaAwesome_States."Exit") -> (x = y?=w20:bool)
  }
  n990 = disable-structure shown="Disabled" {
    disable-tunnel: w2 -> [w1721 _]
    frame Disabled {
      n991 = call "Close LabView?"("Enable"=w1721) -> ("OK"=w1720:bool)  [unwired: 17 in, 1 out]
      n992 = Quit LabVIEW(quit? (T)=w1720) -> ()
    }
    frame Enabled {
    }
  }
